vi "BeamProfiler.vi"() -> ()   [LabVIEW 2015]
uses:
  <vilib>/vision/Image Controls.llb/IMAQ Image.ctl
  <vilib>/userdefined/High Color/IMAQdx.ctl
  <vilib>/vision/driver/IMAQdx.llb/IMAQdx Buffer Number Mode.ctl
  <vilib>/vision/driver/IMAQdx.llb/IMAQdx Acquisition Mode.ctl
  <vilib>/vision/NI_Vision_Development_Module.lvlib
  <vilib>/vision/driver/NI_Vision_Acquisition_Software.lvlib
  <resource>/objmgr/imaqdx.rc
panel:
  out "Histogram Report 2":T1
  in  "Pixel Size":cluster{"X Step":sgl, "Y Step":sgl}={"X Step"=5.2, "Y Step"=5.2} {"Y Step" format="%.2f"; "X Step" format="%.2f"}
  out "Fit Pixel":dbl[](array[numeric])
  out "Ellipse Points":cluster{"x out":dbl, "y out":dbl}[](array[cluster])
  out "Cross lines":T2
  out "ROI Width":dbl
  out "Subsampling":i32(ring)=16 items=["1"=1, "2"=2, "4"=4, "8"=8, "16"=16]
  out "error Fitting":errorcluster
  out "GausFit Time":u32(graph)
  out "Gaus Param":T3(graph)
  in  "Rangefactor \n(multiple of w)":dbl=3.0
  out "Fitting error: Message":string
  out "parameter \narray":dbl[][](array[numeric])
  out "residue":dbl
  out "number of \nfunction calls":i32
  out "Fitting Time \n(ms)":u32
  in  "Gaussianfit":bool
  out "Image to fit":T4(plugin-control)
  in  "Tab Control":T5(tab)
  out "Histogramm of ROI":u32[](graph)
  out "Gray Level Intensities":T6 {"Standard  Deviation" format="%.2f"; "Mean Intensity" format="%.2f"; "Maximum Intensity" format="%.2f"; "Minimum Intensity" format="%.2f"}
  out "Sättigung":dbl format="%.2f %"
  out "3D Image 2":T4(plugin-control)
  in  "3D options":T7={"alpha"=15.0, "beta"=30.0, "border"=20, "background"=85, "plane"=2} {"beta" min=15 max=45 format="%.2f"; "alpha" min=15 max=45 format="%.2f"}
  out "Differece Image to Ideal Gaussian":T4(plugin-control)
  in  "DualZoom":bool
  in  "Show Difference Image":bool
  out "Minimal Value":sgl
  out "Maximal Value":sgl
  out "AbsDiff":T4(plugin-control)
  in  "Show Abs Difference Image":bool
  out "Histogram Diff ROI":T1 {"Standard  Variation" format="%.2f"; "Mean Value" format="%.2f"; "Interval Width" format="%.2f"; "Starting Value" format="%.2f"; "Maximal Value" format="%.2f"; "Minimal Value" format="%.2f"}
  out "Histogram Img ROI":T1 {"Standard  Variation" format="%.2f"; "Mean Value" format="%.2f"; "Interval Width" format="%.2f"; "Starting Value" format="%.2f"; "Maximal Value" format="%.2f"; "Minimal Value" format="%.2f"}
  out "Integrated Pixels":cluster{sgl, sgl}(graph)
  out "AbsDiff/Imag":sgl(graph)
  out "AbsDifference/ImageSum":sgl
  out "Integrated AbsDiff":sgl
  out "Integrated CamImage":sgl
  out "Recorded Background":T4(plugin-control)
  out "iValue\nChart":dbl(graph)
  in  "soll":dbl=220.0 min=10.0 max=240.0 step=1.0
  out "iValue":dbl
  in  "1/T":dbl=4.0
  out "ist":dbl
  out "ImgMax/Max":dbl
  in  "AutoAcquisitionState":T8(ring)
  in  "Next AEC & AGC\niteration":bool
  in  "Enable AEC & AGC":bool
  in  "Max Intensity":dbl=250.0 max=254.0
  out "Time\nAGC\nHist":dbl
  out "Time\nAGC/AEC\ncycle":dbl
  out "State":sgl(graph)
  in  "Gaussian Fit completed":bool
  out "Exit from Target Point":bool
  out "Beam Parameters Target Point":T9
  out "Target Point cross lines":T2
  out "Target Points Ellipse Points":cluster{"x out":dbl, "y out":dbl}[](array[cluster])
  in  "Set Target Point":bool
  in  "Show Target \nPoint Axes":bool
  out "Start StreamingLED":bool
  out "AcquisitionTime":dbl(graph)
  out "Time\nAcqisition(s)":dbl
  out "Time\nEvent(ms)":u32
  out "Histogram Report":T1
  out "Exit from AGC/AEC":bool
  out "ActValue:InverseExposure":dbl format="1 / %#_g ms"
  out "Image Busy":bool
  in  "Show Axes Overlay":bool=TRUE
  out "Exit from stream complete":bool
  out "Exit from Control refresh":bool
  out "Exit from Gaussian cycle":bool
  out "Exit from Eventloop":bool
  out "image heigth":u16
  out "image width":u16
  in  "Resolution":cluster{"X Step":u16, "Y Step":u16}={"X Step"=1280, "Y Step"=1024}
  out "IMAQ Actual Image":T4(plugin-control)
  out "GValueMin":dbl format="%#_4g"
  out "GValueMax":dbl format="%#_4g"
  out "EValueMin":dbl format="%#_4g"
  out "EValueMax":dbl format="%#_4g"
  out "error\nControl\nrefresh":errorcluster
  out "Buffer Number":u32
  out "Frame Rate":dbl(knob) scale=0.0..20.0
  out "ActVal:Gain":string
  out "ActValue:Exposure":string
  in  "Gain::Mode":u32(ring)=2 caption="Exposure::Mode" items=["Auto (Extended)", "Auto (Standard)", "Manual"]
  in  "Exposure::Mode":u32(ring)=2 items=["Auto (Extended)", "Auto (Standard)", "Manual"]
  in  "Set Gain":bool
  in  "Set Exposure":bool
  in  "Set: Gain::Value":i64 caption="Gain::Value" min=0 max=1728 step=16
  in  "Set: Exposure::Value":dbl=0.0625 caption="Exposure::Value" min=0.0001220703125 max=0.125
  out "Camera Handle":T10 caption="Session Out"
  in  "Camera Name":refnum<k21>="cam0" caption="IMAQdx Session"
  out "IMAQ Actual Image (RGB)":T4
  in  "Cyclic\nCalculation":bool=TRUE
  in  "Cycletime Task\nGaussian Fit":u32=1000
  out "Stream completed":bool
  in  "Stop Streaming":bool
  in  "Start Streaming":bool
  out "Stream error out":errorcluster
  out "Streaming Started":bool
  out "IMAQ Background Image":T4
  in  "Subtract Background":bool
  in  "Record Background":bool
  out "CAM\ninitialized":bool
  in  "Direction (NW)":T11(ring)
  in  "3D Image":bool
  in  "CalcHistogram":bool
  out "EventState":string
  out "error Event":errorcluster
  in  "error in":errorcluster
  in  "Start":bool
  in  "Tab Beam":enum32{"Beam Parameters", "Navigate to Target"}(tab)
  out "Beam Parameters":T9 {"Amplitude (Counts)" format="%#.2f"; "Position X (µm)" format="%.2f"; "Position Y (µm)" format="%.2f"; "Width 1 (µm)*" format="%.2f"; "Width 2 (µm)*" format="%.2f"; "Angle (°)" format="%.2f"; "Offset (Counts)" format="%.2f"}
  out "Mean \nRadius":dbl
  out "Ellipticity":dbl format="%#_3g"
  out "Point":T12 {"Y" format="%.2f"; "X" format="%.2f"}
  in  "Threshold (µm)":dbl=52.0
  out "dy":dbl
  out "dx":dbl
  out "left":bool
  out "down":bool
  out "up":bool
  out "right":bool
  out "center":bool
  out "Beam Parameters\nfor Target":T13
  out "Absolute Distance (µm)":dbl
  in  "stop":bool
  # "Shutdown"
  # "Overview: .\nRequirements: Vision Development Software, Vision Acquisition Software.\nInstructions: \n1. Select 'Camera Name',  'Resolution' and 'Pixel Size'\n2. Run the VI.\n3. Press 'Start'\n4. Pausing/Resuming Image with Start/Stop Streaming\n\nExit with 'Stop'"
  # "Aquisition Settings"
  # "ms"
  # "x /µm"
  # "y /µm"
  # "ms"
  # "Guess Pixel"
  # "Fit RAW"
  # "Fit Pixel"
  # "Fit µm"
  # "Amplitude"
  # "Position Mean X"
  # "Position Mean Y"
  # "Width 1 (1/e)"
  # "Width 2(1/e)"
  # "Orient. Angle"
  # "Offset"
  # "w(1/e) *sqrt(2) = w(1/e^2)"
  # "x"
  # "µm"
  # "Note: ROI has to be selected"
  # "Note: \nDifferent color scale"
  # "Background:\n1. Turn off subtraction\n2. Hide beam\n3. Take Image (Stream)\n4. Record background\nNote: not compatible \nwith AutoExposure"
  # "x"
  # "pixels"
  # "* Radius, 1/e^2, 13,5%, Width 1 > Width 2"
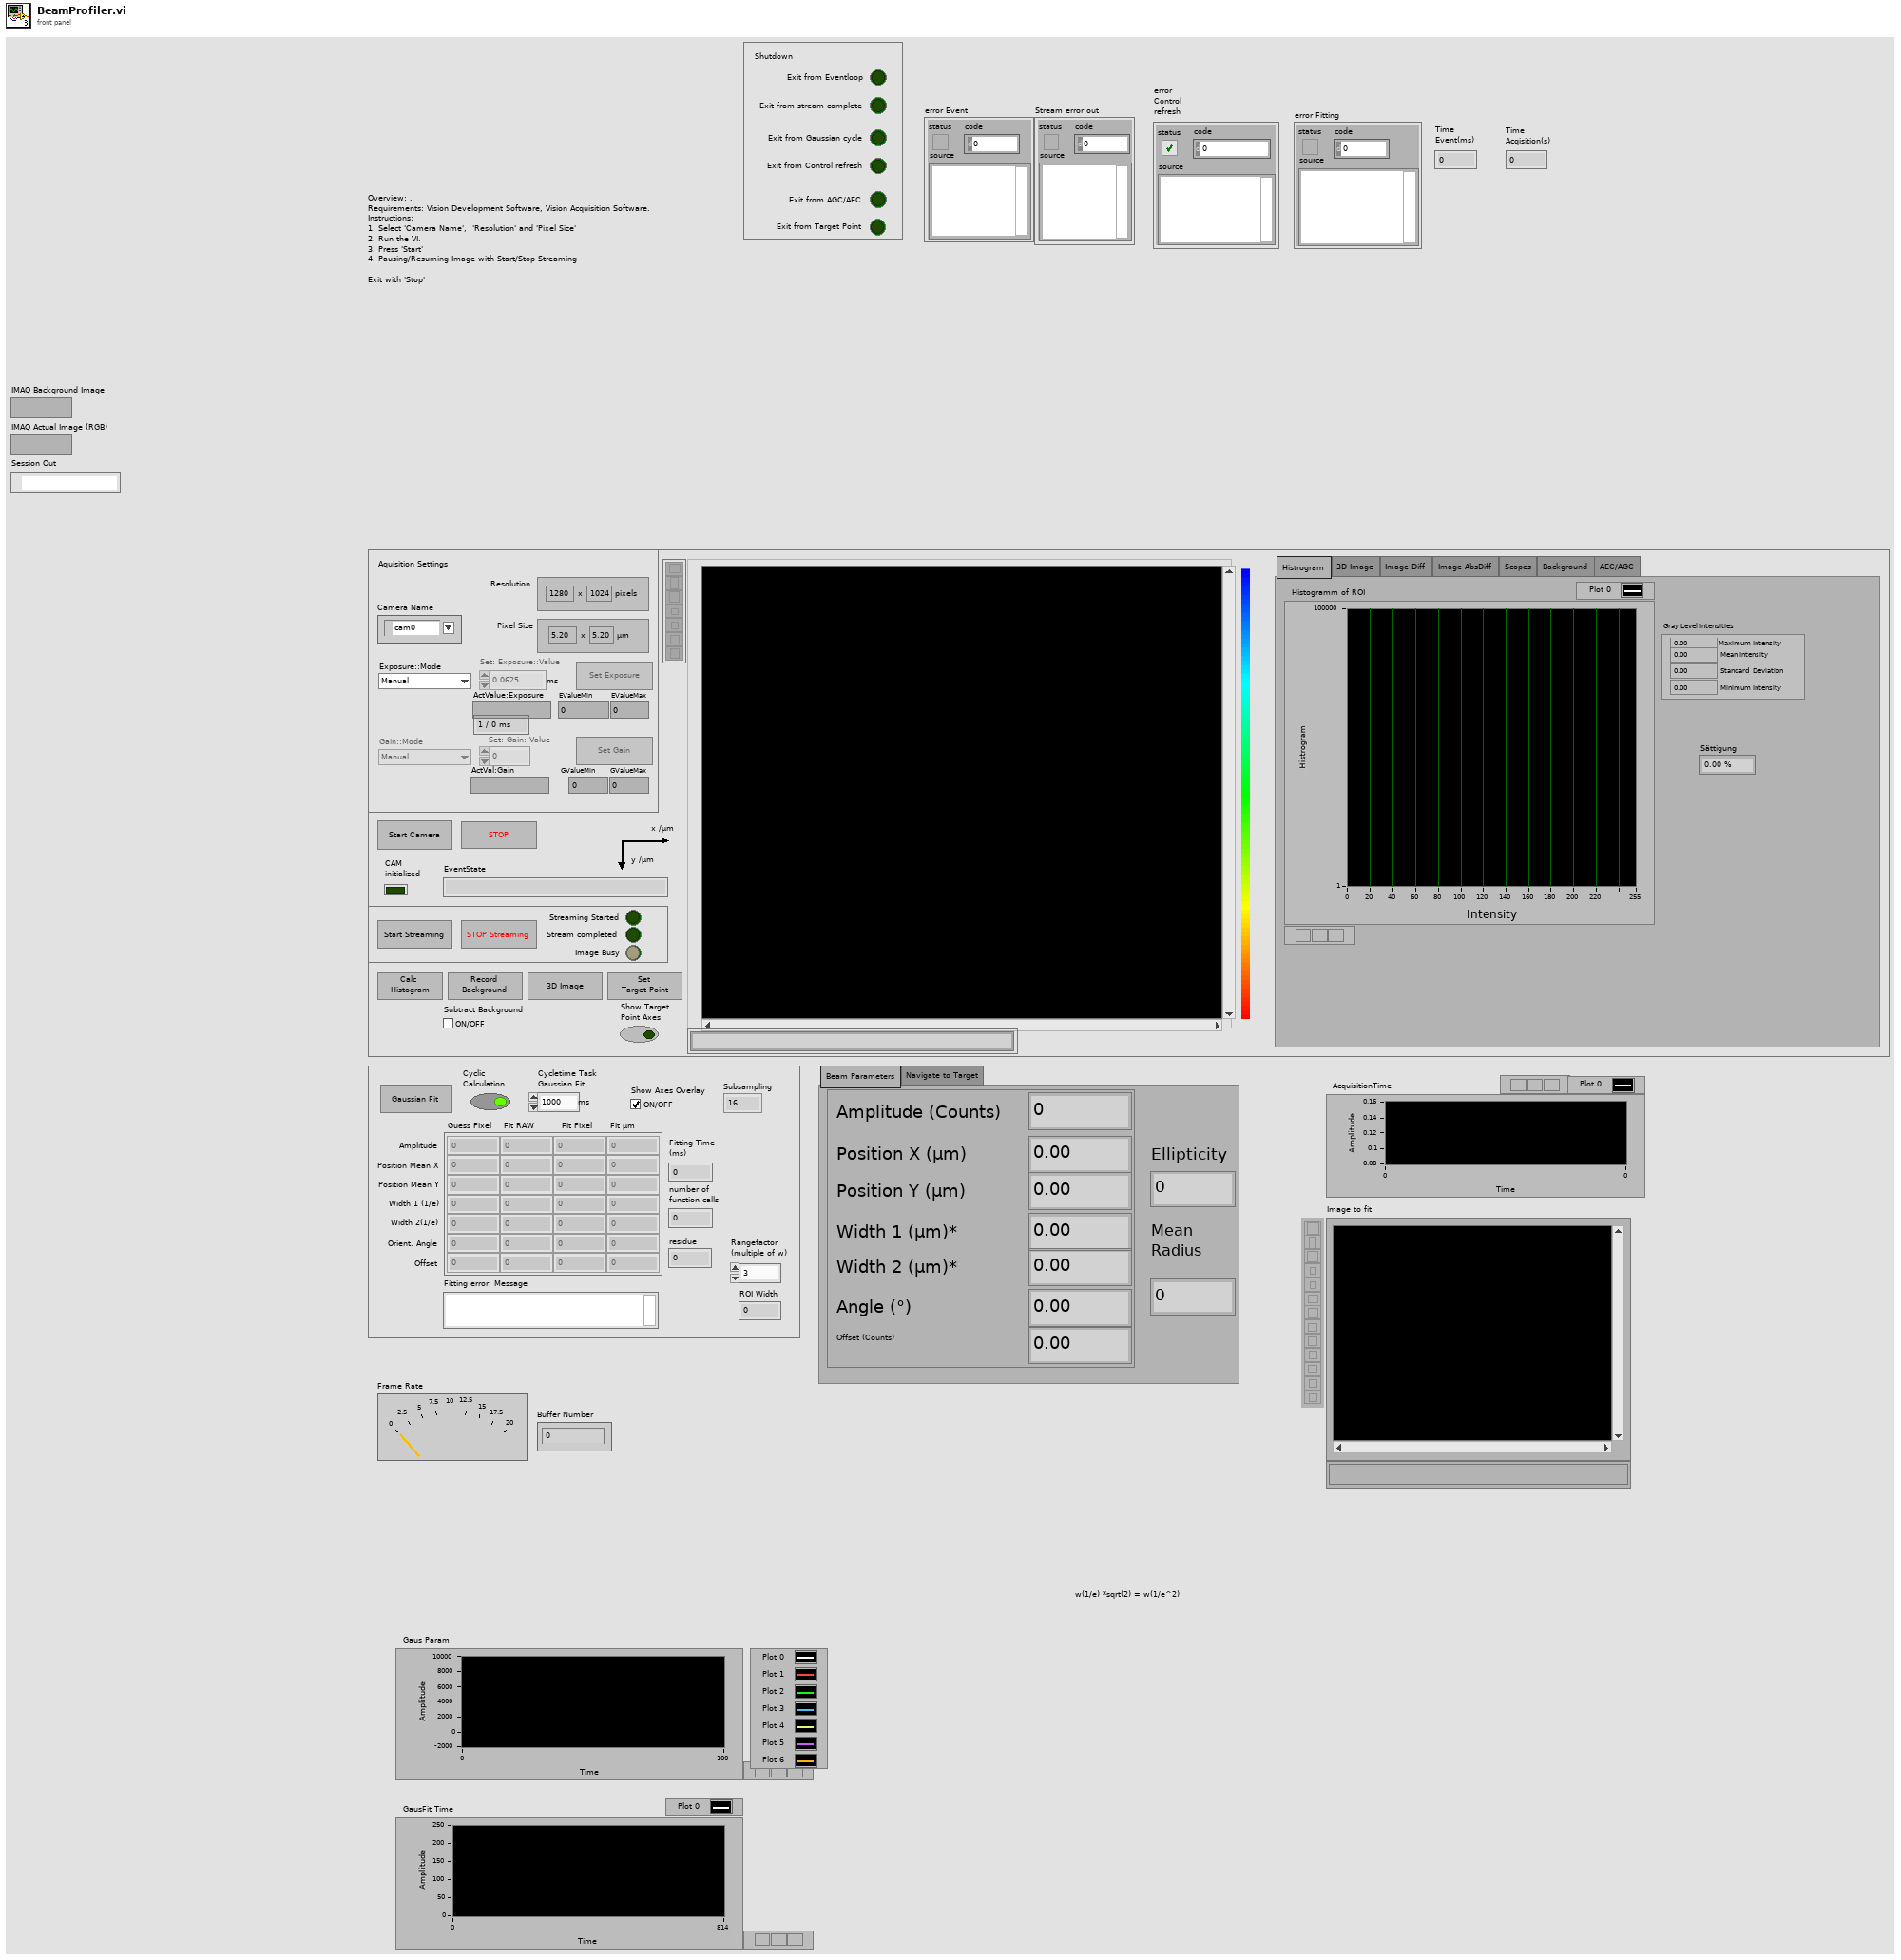
[diagram p1: front panel]
types:
  T1 = cluster{"histogram":u32[], "Minimal Value":sgl, "Maximal Value":sgl, "Starting Value":sgl, "Interval Width":sgl, "Mean Value":sgl, "Standard  Variation":sgl, "Area (pixels)":i32}
  T2 = cluster{"Line1 Start Point":cluster{"X":i32, "Y":i32}, "Line1 End Point":cluster{"X":i32, "Y":i32}, "Line2 Start Point":cluster{"X":i32, "Y":i32}, "Line2 End Point":cluster{"X":i32, "Y":i32}}
  T3 = cluster{"Amplitude (Counts)":dbl, "Position Max X(µm)":dbl, "Position Max Y(µm)":dbl, "Width 1 (µm)":dbl, "Width 2 (µm)":dbl, "Angle (°)":dbl, "Offset (Counts)":dbl}
  T4 = typedef "IMAQ Image.ctl" = refnum<image>
  T5 = enum32{"Histrogram", "3D Image", "Image Diff", "Image AbsDiff", "Scopes", "Background", "AEC/AGC"}
  T6 = cluster{"Mean Intensity":sgl, "Standard  Deviation":sgl, "Minimum Intensity":sgl, "Maximum Intensity":sgl}
  T7 = cluster{"alpha":sgl, "beta":sgl, "border":i32, "background":i32, "plane":i32}
  T8 = enum16{"idle", "init", "Wait before exposure", "Find max exposure", "Wait before gain", "Find max gain"}
  T9 = cluster{"Amplitude (Counts)":dbl, "Position X (µm)":dbl, "Position Y (µm)":dbl, "Width 1 (µm)*":dbl, "Width 2 (µm)*":dbl, "Angle (°)":dbl, "Offset (Counts)":dbl}
  T10 = typedef "IMAQdx.ctl" = refnum<k21>
  T11 = enum32{"North West", "South West", "South East", "North East"}
  T12 = typedef "IMAQ Point" = cluster{"X":sgl, "Y":sgl}
  T13 = cluster{"Amplitude (Counts)":dbl, "Position X (µm)":dbl, "Position Y (µm)":dbl}
  T14 = typedef "Image Type" = u32
  T15 = cluster{"Global Rectangle":i32[], "Contours":cluster{"Contour Type":u32, "ROI Type":u32, "Points":i32[]}[]}
  T16 = enum8{"Enabled", "Disabled", "Disabled and Grayed Out"}
  T17 = enum32{"Histrogram", "3D Image", "Image Diff", "Image AbsDiff", "Scopes", "Background"}
  T18 = typedef "NI_Vision_Acquisition_Software.lvlib/IMAQdx Acquisition Mode.ctl" = enum32{"One Shot", "Continuous"}
  T19 = cluster{"Amplitude (Counts)":dbl, "Position Max X(µm)":dbl, "Position Max Y(µm)":dbl}
  T20 = typedef "NI_Vision_Acquisition_Software.lvlib/IMAQdx Buffer Number Mode.ctl" = enum32{"Next", "Last", "Buffer Number", "Every", "Last New"}
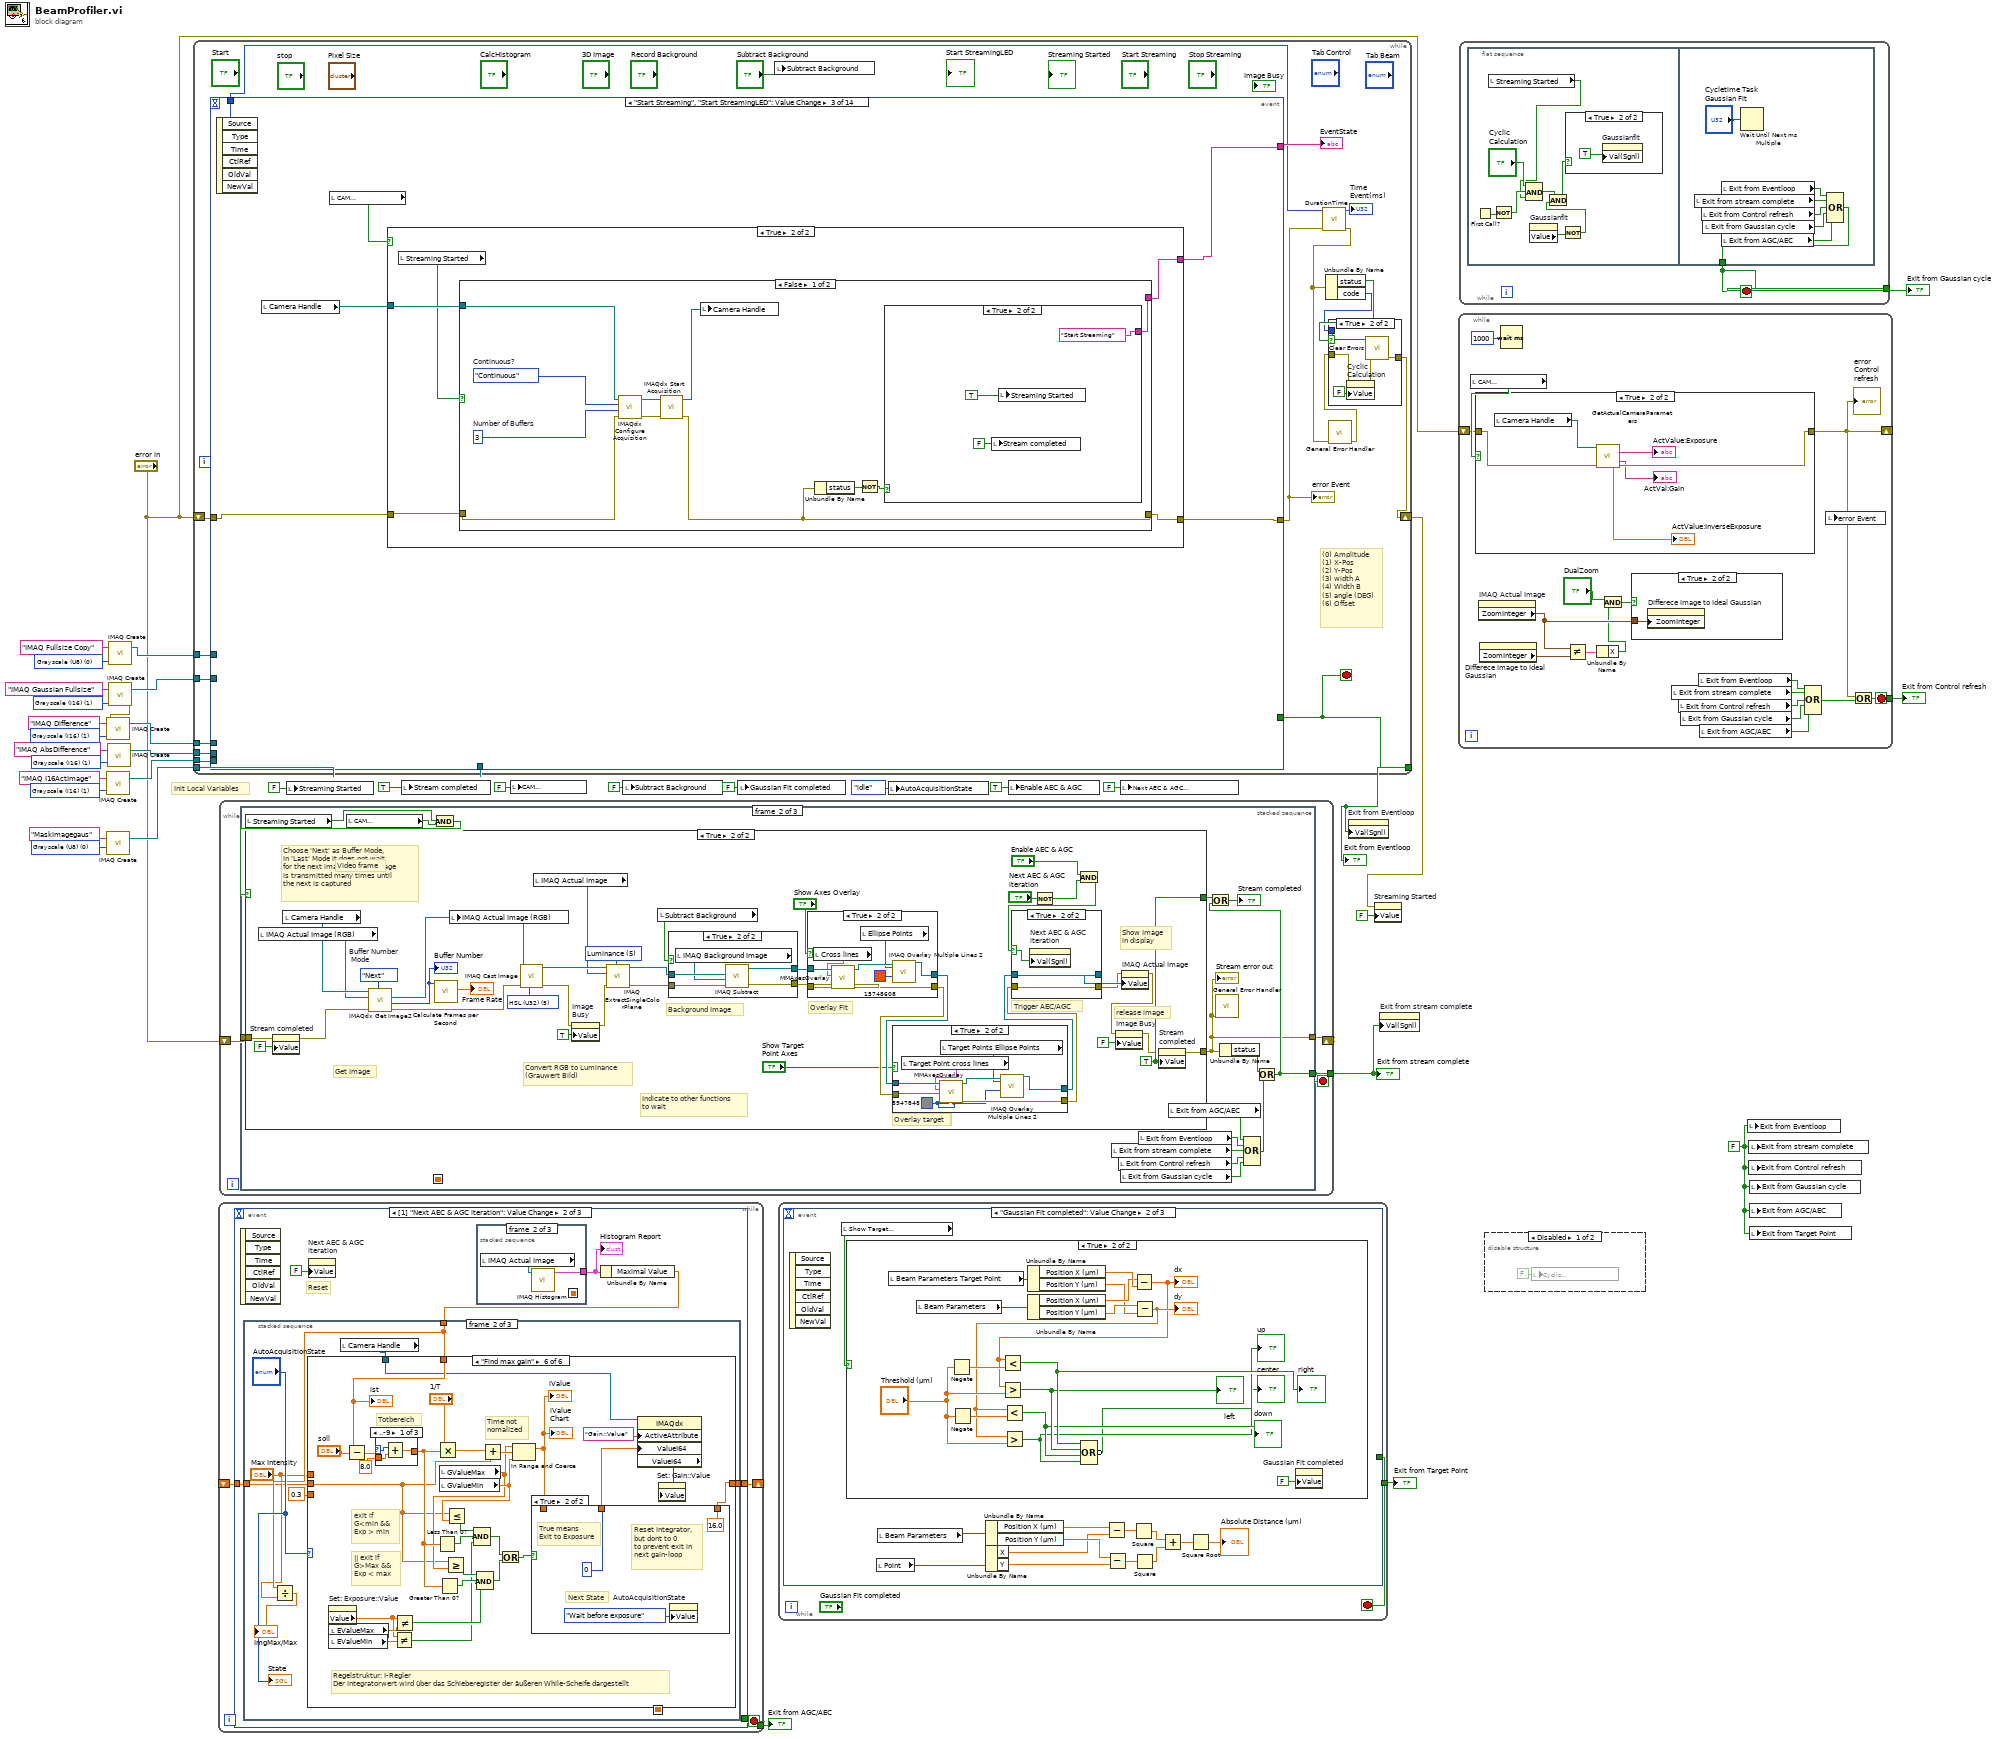
[diagram p0: block diagram]
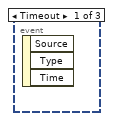
[diagram p2: hidden frame]
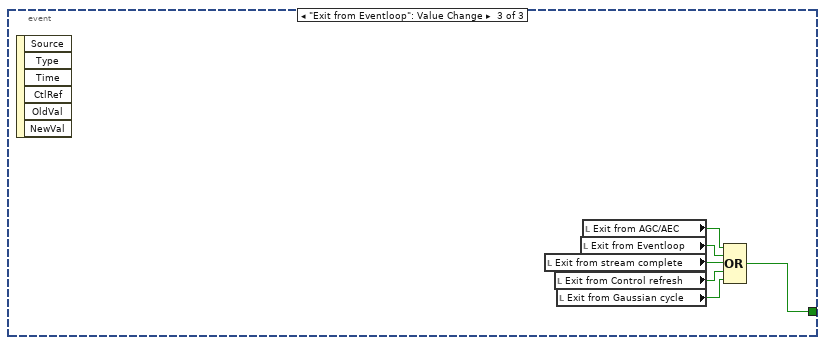
[diagram p4: hidden frame]
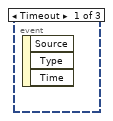
[diagram p6: hidden frame]
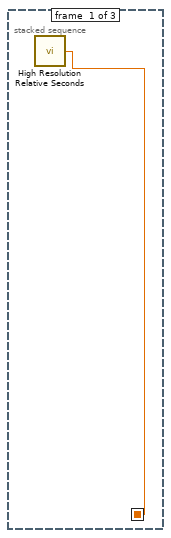
[diagram p7: hidden frame]
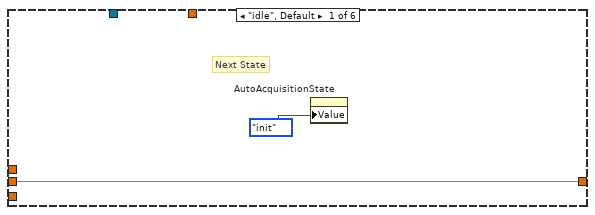
[diagram p8: hidden frame]
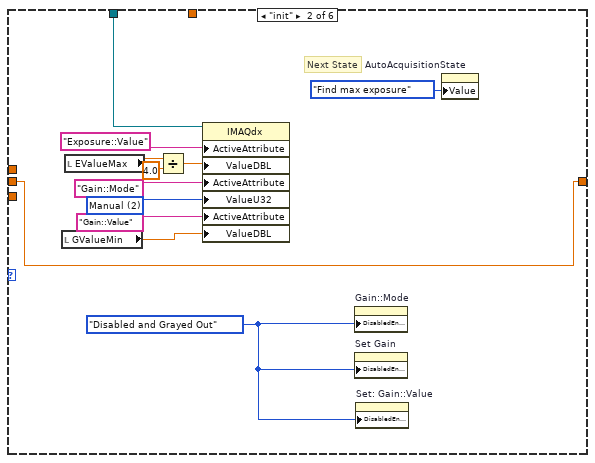
[diagram p9: hidden frame]
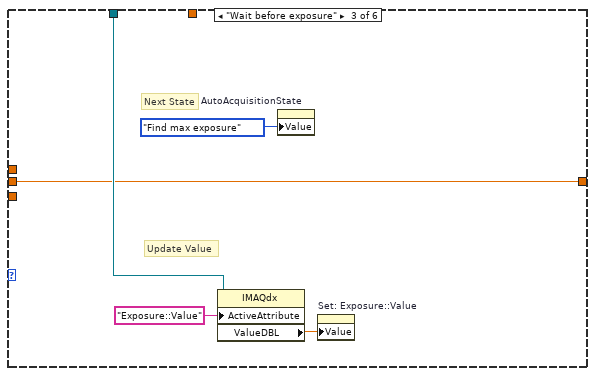
[diagram p10: hidden frame]
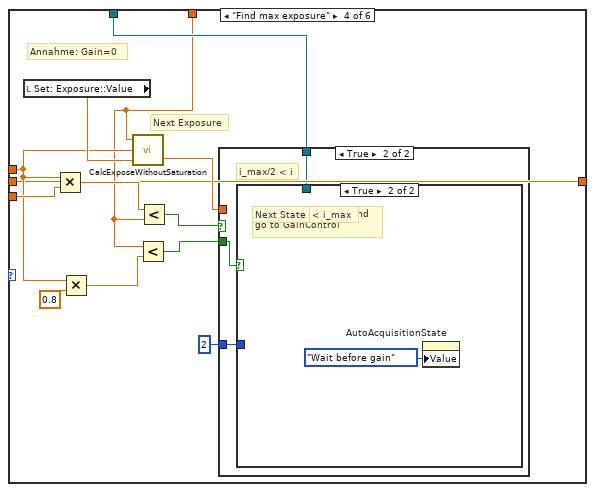
[diagram p11: hidden frame]
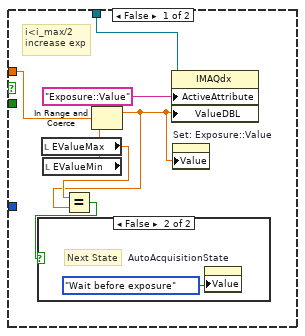
[diagram p12: hidden frame]
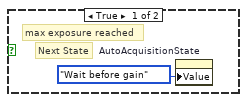
[diagram p13: hidden frame]
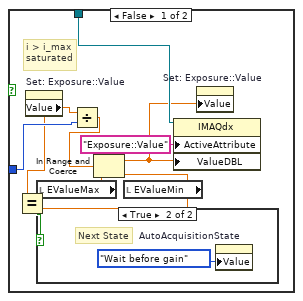
[diagram p14: hidden frame]
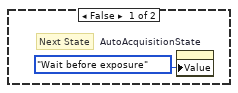
[diagram p15: hidden frame]
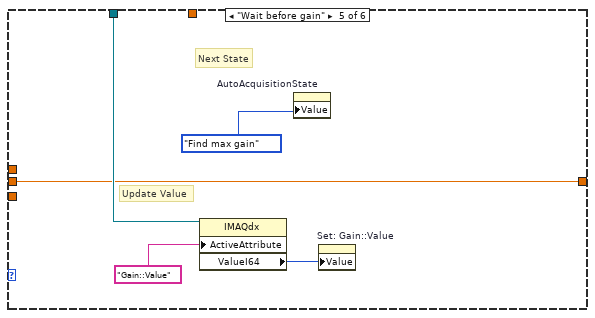
[diagram p16: hidden frame]
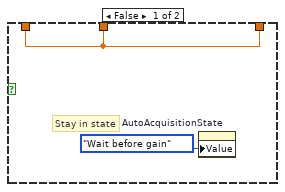
[diagram p17: hidden frame]
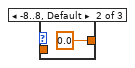
[diagram p18: hidden frame]
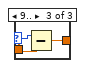
[diagram p19: hidden frame]
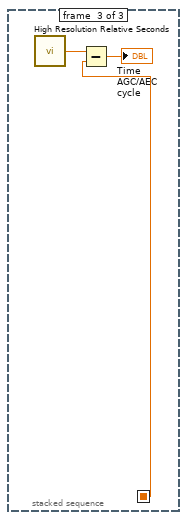
[diagram p20: hidden frame]
diagram:
  w3 = T14 0 items=["Grayscale (U8)", "Grayscale (I16)", "Grayscale (SGL)", "Complex (CSG)", "RGB (U32)", "HSL (U32)", "RGB (U64)", "Grayscale (U16)"] ("Image Type")
  w5 = T14 0 items=["Grayscale (U8)", "Grayscale (I16)", "Grayscale (SGL)", "Complex (CSG)", "RGB (U32)", "HSL (U32)", "RGB (U64)", "Grayscale (U16)"] ("Image Type")
  w9 = T14 1 items=["Grayscale (U8)", "Grayscale (I16)", "Grayscale (SGL)", "Complex (CSG)", "RGB (U32)", "HSL (U32)", "RGB (U64)", "Grayscale (U16)"] ("Image Type")
  w20 = T14 1 items=["Grayscale (U8)", "Grayscale (I16)", "Grayscale (SGL)", "Complex (CSG)", "RGB (U32)", "HSL (U32)", "RGB (U64)", "Grayscale (U16)"] ("Image Type")
  w16 = T14 1 items=["Grayscale (U8)", "Grayscale (I16)", "Grayscale (SGL)", "Complex (CSG)", "RGB (U32)", "HSL (U32)", "RGB (U64)", "Grayscale (U16)"] ("Image Type")
  w15 = T14 1 items=["Grayscale (U8)", "Grayscale (I16)", "Grayscale (SGL)", "Complex (CSG)", "RGB (U32)", "HSL (U32)", "RGB (U64)", "Grayscale (U16)"] ("Image Type")
  w22 = FALSE ("Gaussianfit")
  # "Init Local Variables"
  n1 = call "IMAQ Create"("Image Name"="IMAQ I16ActImage", "Image Type"=w9) -> ("New Image"=w8:T4)  [unwired: 3 in, 1 out]
  n2 = call "IMAQ Create"("Image Name"="MaskImagegaus", "Image Type"=w5) -> ("New Image"=w6:T4)  [unwired: 3 in, 1 out]
  n3 = call "IMAQ Create"("Image Name"="IMAQ AbsDifference", "Image Type"=w20) -> ("New Image"=w11:T4)  [unwired: 3 in, 1 out]
  n4 = call "IMAQ Create"("Image Name"="IMAQ Gaussian Fullsize", "Image Type"=w15) -> ("New Image"=w13:T4, "error out"=w18:errorcluster)  [unwired: 3 in]
  n5 = call "IMAQ Create"("Image Name"="IMAQ Difference", "Image Type"=w16, "error in (no error)"=w18) -> ("New Image"=w12:T4)  [unwired: 2 in, 1 out]
  n6 = call "IMAQ Create"("Image Name"="IMAQ Fullsize Copy", "Image Type"=w3) -> ("New Image"=w2:T4)  [unwired: 3 in, 1 out]
  n7 = while {
    shift-right: [w51] -> w33
    shift-left: "error in" -> [w53]
    tunnel: [w39] -> w27
    tunnel: w13 -> [w44]
    tunnel: w12 -> [w43]
    tunnel: w11 -> [w42]
    tunnel: w8 -> [w41]
    tunnel: w6 -> [w38]
    tunnel: w2 -> [w40]
    stop <- w39 stop-if-true
    # "(0) Amplitude\n(1) X-Pos\n(2) Y-Pos\n(3) width A\n(4) Width B\n(5) angle (DEG)\n(6) Offset"
    n8 = event shown="[2] \"Start Streaming\", \"Start StreamingLED\": Value Change" {
      selector: _ -> [_ _ _ _ _ _ _ _ _ _ _ _ _ _]
      dyn-events: _ -> [_ _ _ _ _ _ _ _ _ _ _ _ _ _]
      timeout: _ -> [_ _ _ _ _ _ _ _ _ _ _ _ _ _]
      tunnel: [_ _ _ _ _ _ _ _ _ _ _ w512 _ _] -> w39
      tunnel: [_ w68 w114 w149 w222 w319 w337 w353 w393 w429 w456 w514 w562 _] -> w45
      tunnel: ["Timeout" ("MainState") w66 w113 w148 _ w320 w336 w350 w390 w427 w457 w508 w561 _] -> w55
      tunnel: w53 -> [_ w65 w112 _ w209 w322 w338 w354 w394 w428 w455 w507 w565 _]
      tunnel: [w62 w64 w111 w141 w212 w318 w334 w352 w392 w426 w454 w506 w564 _] -> w49
      tunnel: w44 -> [_ _ _ _ w189 _ _ _ _ _ _ _ _ _]
      tunnel: w43 -> [_ _ _ _ w185 _ _ _ _ _ _ _ _ _]
      tunnel: w42 -> [_ _ _ _ w186 _ _ _ _ _ _ _ _ _]
      tunnel: w41 -> [_ _ _ _ w187 _ _ _ _ _ _ _ _ _]
      tunnel: w40 -> [_ _ _ _ w234 _ _ _ _ _ _ _ _ _]
      tunnel: w38 -> [_ _ _ _ w188 _ _ _ _ _ _ _ _ _]
      event Timeout {
        n9 = event-data() -> ("Time"=w62:u32)  [unwired: 1 in, 2 out]
      }
      event "Start": Value Change {
        n10 = event-data() -> ("Time"=w64:u32)  [unwired: 1 in, 5 out]
        n11 = local read "CAM\ninitialized"() -> (w67:bool)
        n12 = case shown="False" w67 {
          tunnel: [w86 w109] -> w68
          tunnel: ["Camera starting" ("MainState") "Camera already started" ("MainState")] -> w66
          tunnel: w65 -> [w90 w109]
          frame False {
            w87 = T14 0 items=["Grayscale (U8)", "Grayscale (I16)", "Grayscale (SGL)", "Complex (CSG)", "RGB (U32)", "HSL (U32)", "RGB (U64)"] ("Image Type")
            w94 = T14 0 items=["Grayscale (U8)", "Grayscale (I16)", "Grayscale (SGL)", "Complex (CSG)", "RGB (U32)", "HSL (U32)", "RGB (U64)"] ("Image Type")
            w96 = T14 0 items=["Grayscale (U8)", "Grayscale (I16)", "Grayscale (SGL)", "Complex (CSG)", "RGB (U32)", "HSL (U32)", "RGB (U64)", "Grayscale (U16)"] ("Image Type")
            n13 = Unbundle By Name("Resolution") -> ("X Step"=→"image width":u16, "Y Step"=→"image heigth":u16)
            n14 = call <vilib>:"IMAQdx Open Camera.vi"("error in"=w90, "Session In"="Camera Name") -> ("error out"=w89:errorcluster, "Session Out"=w85:T10)  [unwired: 1 in, 7 out]
            "Camera Handle" <- w85
            n15 = call "IMAQ Create"("Image Name"="Actual Image", "Image Type"=w96, "error in (no error)"=w89) -> ("New Image"=w78:T4, "error out"=w92:errorcluster)  [unwired: 2 in]
            "IMAQ Actual Image" <- w78
            n16 = call "IMAQ Create"("Image Name"="Actual Image (RGB)", "Image Type"=w94, "error in (no error)"=w92) -> ("New Image"=w93:T4, "error out"=w91:errorcluster)  [unwired: 2 in]
            "IMAQ Actual Image (RGB)" <- w93
            n17 = call "IMAQ Create"("Image Name"="Background Image", "Image Type"=w87, "error in (no error)"=w91) -> ("New Image"=w99:T4, "error out"=w81:errorcluster)  [unwired: 2 in]
            "IMAQ Background Image" <- w99
            n18 = local write "Camera Handle"(w85) -> ()
            n19 = local write "IMAQ Actual Image (RGB)"(w93) -> ()
            n20 = local write "IMAQ Background Image"(w99) -> ()
            n21 = local write "IMAQ Actual Image"(w78) -> ()
            n22 = disable-structure shown="Enabled" {
              disable-tunnel: w81 -> [w107 _]
              disable-tunnel: [w106 _] -> w80
              frame Enabled {
                w105 = u32 0 items=["Auto (Extended)", "Auto (Standard)", "Manual"] ("Gain::Mode")
                n23 = property on="Exposure::Mode" class="Ring (strict)"(error in=w107, "Val(Sgnl)"=w105) -> (error out=w108:errorcluster)  [unwired: 1 in, 1 out]
                n24 = property on="Gain::Mode" class="Ring (strict)"(error in=w108, "Val(Sgnl)"=w105) -> (error out=w106:errorcluster)  [unwired: 1 in, 1 out]
              }
              frame Disabled {
              }
            }
            n25 = property class="IMAQdx"(reference=w85, error in=w80, "ActiveAttribute"="Exposure::Value", "ActiveAttribute"="Gain::Value") -> (error out=w86:errorcluster, "ValueDBL"=w83:dbl, "MinDBL"=w74:dbl, "MaxDBL"=w73:dbl, "ValueI64"=w79:i64, "MinDBL"=w72:dbl, "MaxDBL"=w71:dbl)  [unwired: 1 out]
            "EValueMin" <- w74
            "EValueMax" <- w73
            "GValueMin" <- w72
            "GValueMax" <- w71
            n26 = property on="Set: Exposure::Value" class="DigNum (strict)"("Value"=w83) -> ()  [unwired: 2 in, 2 out]
            n27 = property on="Set: Gain::Value" class="DigNum (strict)"("Value"=w79) -> ()  [unwired: 2 in, 2 out]
            n28 = property on="Set: Gain::Value" class="DigNum (strict)"("Maximum"=w71, "Minimum"=w72) -> ()  [unwired: 2 in, 2 out]
            n29 = property on="Set: Exposure::Value" class="DigNum (strict)"("Minimum"=w74, "Maximum"=w73) -> ()  [unwired: 2 in, 2 out]
            n30 = Unbundle By Name(w86) -> ("status"=w98:bool)
            n31 = Not(x=w98) -> (.not. x?=w97:bool)
            n32 = Or(x=TRUE, y=w97) -> (x .or. y?=→"CAM\ninitialized":bool)
            n33 = property on="Start StreamingLED" class="Bool (strict)"() -> ("Value"=w70:bool)  [unwired: 2 in, 2 out]
            n34 = Not(x=w70) -> (.not. x?=w69:bool)
            n35 = property on="Start StreamingLED" class="Bool (strict)"("Val(Sgnl)"=w69) -> ()  [unwired: 2 in, 2 out]
          }
          frame True {
          }
        }
      }
      event "Start Streaming", "Start StreamingLED": Value Change {
        n36 = event-data() -> ("Time"=w111:u32)  [unwired: 1 in, 5 out]
        n37 = local read "Camera Handle"() -> (w116:T10)
        n38 = local read "CAM\ninitialized"() -> (w115:bool)
        n39 = case shown="True" w115 {
          tunnel: w116 -> [_ w122]
          tunnel: w112 -> [w118 w121]
          tunnel: [w118 w120] -> w114
          tunnel: ["Camera not initialized, Press Start Camera" ("MainState") w123] -> w113
          frame False {
            n40 = call "Display Message to User2"() -> ()  [unwired: 10 in, 2 out]
          }
          frame True {
            n41 = local read "Streaming Started"() -> (w119:bool)
            n42 = case shown="False" w119 {
              tunnel: [w132 "Stream already started" ("MainState")] -> w123
              tunnel: w122 -> [w129 _]
              tunnel: w121 -> [w126 w139]
              tunnel: [w125 w139] -> w120
              frame False {
                w127 = u32 3  # Number of Buffers
                w128 = IMAQdx_Acquisition_Mode."Continuous"  # Continuous?
                n43 = call <vilib>:"IMAQdx Configure Acquisition.vi"("error in"=w126, "Number of Buffers"=w127, "Continuous?"=w128, "Session In"=w129) -> ("error out"=w131:errorcluster, "Session Out"=w130:T10)  [unwired: 6 out]
                n44 = call <vilib>:"IMAQdx Start Acquisition.vi"("error in"=w131, "Session In"=w130) -> ("error out"=w125:errorcluster, "Session Out"=w124:T10)  [unwired: 8 out]
                n45 = local write "Camera Handle"(w124) -> ()
                n46 = Unbundle By Name(w125) -> ("status"=w134:bool)
                n47 = Not(x=w134) -> (.not. x?=w133:bool)
                n48 = case shown="True" w133 {
                  tunnel: ["Error while starting stream" ("MainState") "Start Streaming" ("MainState")] -> w132
                  frame False {
                  }
                  frame True {
                    n49 = local write "Stream completed"(FALSE ("Stream completed")) -> ()
                    n50 = local write "Streaming Started"(TRUE ("Stream Start")) -> ()
                  }
                }
              }
              frame True {
              }
            }
          }
        }
      }
      event "Stop Streaming": Value Change {
        n51 = event-data() -> ("Time"=w141:u32)  [unwired: 1 in, 5 out]
        n52 = local read "Streaming Started"() -> (w151:bool)
        n53 = local read "Camera Handle"() -> (w152:T10)
        n54 = local read "error Event"() -> (w150:errorcluster)
        n55 = flat-sequence {
          tunnel: w150 -> [w154]
          tunnel: w151 -> [w155]
          tunnel: w152 -> [w156]
          tunnel: [w156] -> w147
          tunnel: [w155] -> w145
          tunnel: [w154] -> w143
          tunnel: w147 -> [w160]
          tunnel: [w160] -> w146
          tunnel: w145 -> [w159]
          tunnel: [w159] -> w144
          tunnel: w143 -> [w158]
          tunnel: [w158] -> w142
          tunnel: [w169] -> w149
          tunnel: [w168] -> w148
          tunnel: w146 -> [w172]
          tunnel: w144 -> [w171]
          tunnel: w142 -> [w170]
          frame #0 {
            n56 = local write "Streaming Started"(FALSE ("Streaming Started")) -> ()
          }
          frame #1 {
            # "With Timeout"
            n57 = Tick Count (ms)() -> (millisecond timer value=w157:u32)
            n58 = while {
              tunnel: w157 -> [w166]
              stop <- w161 stop-if-true
              n59 = local read "Stream completed"() -> (w162:bool)
              n60 = Tick Count (ms)() -> (millisecond timer value=w167:u32)
              n61 = Subtract(x=w167, y=w166) -> (x-y=w165:u32)
              n62 = Greater?(x=w165, y=u32 2000) -> (0:w163:bool)
              n63 = Or(x=w162, y=w163) -> (x .or. y?=w161:bool)
            }
          }
          frame #2 {
            n64 = case shown="True" w171 {
              tunnel: w172 -> [_ w176]
              tunnel: w170 -> [w174 w178]
              tunnel: [w174 w177] -> w169
              tunnel: ["no stream running" ("MainState") "stream stopped" ("MainState")] -> w168
              frame False {
              }
              frame True {
                n65 = call <vilib>:"IMAQdx Stop Acquisition.vi"("error in"=w178, "Session In"=w176) -> ("error out"=w179:errorcluster, "Session Out"=w180:T10)  [unwired: 8 out]
                n66 = call <vilib>:"IMAQdx Unconfigure Acquisition.vi"("error in"=w179, "Session In"=w180) -> ("error out"=w177:errorcluster, "Session Out"=w175:T10)  [unwired: 8 out]
                n67 = local write "Camera Handle"(w175) -> ()
              }
            }
          }
        }
      }
      event "Gaussianfit": Value Change {
        # "Der Fehler wird gesondert\nangzeigt und nach einem \nZyklus gelöscht"
        # "Difference Image"
        # "Todo: Possibility to deactivate AutoRoi"
        # "Previous"
        # "Indicator for Target finding \ncycle"
        n68 = event-data() -> ("Time"=w212:u32)  [unwired: 1 in, 5 out]
        n69 = Or(x="Show Difference Image", y="Show Abs Difference Image") -> (x .or. y?=w184:bool)
        n70 = flat-sequence {
          tunnel: w234 -> [w317]
          tunnel: w233 -> [w316]
          tunnel: [w315] -> w217
          tunnel: w209 -> [w314]
          tunnel: [w313] -> w208
          frame #0 {
            n71 = while {
              stop <- w312 continue-if-true
              n72 = property on="Image Busy" class="Bool (strict)"() -> ("Value"=w312:bool)  [unwired: 2 in, 2 out]
            }
          }
          frame #1 {
            n73 = call "IMAQ Copy"("error in (no error)"=w314, "Image Dst"=w317, "Image Src"=w316) -> ("error out"=w313:errorcluster, "Image Dst Out"=w315:T4)  [unwired: 3 in]
          }
        }
        n74 = local read "IMAQ Actual Image"() -> (w233:T4)
        n75 = local read "error Fitting"() -> (w195:errorcluster)
        n76 = local read "residue"() -> (w199:dbl)
        n77 = local read "Fit Pixel"() -> (w197:dbl[])
        n78 = Unbundle By Name(w195) -> ("status"=w194:bool, "code"=w196:i32)
        n79 = case shown="True" w194 {
          tunnel: w196 -> [_ w300]
          tunnel: w195 -> [_ w299]
          frame False {
          }
          frame True {
            n80 = call <vilib>:"Clear Errors.vi"("error in (no error)"=w299, "specific error code to clear (0: all)"=w300) -> ()  [unwired: 4 in, 2 out]
          }
        }
        n81 = First Call?() -> (First Call?: T/F=w201:bool)
        n82 = Equal To 0?(x=w199) -> (x = 0?=w200:bool)
        n83 = Greater?(x=w199, y=100.0) -> (0:w202:bool)
        n84 = local read "Resolution"() -> (w193:cluster{"X Step":u16, "Y Step":u16})
        n85 = Compound Arithmetic op=OR(w202, w200, w201, w194) -> (w198:bool)
        n86 = case shown="True" w198 {
          tunnel: [w302 w306] -> w190
          tunnel: w217 -> [_ w305]
          tunnel: w208 -> [w301 w304]
          tunnel: [w301 w303] -> w207
          tunnel: w197 -> [w302 _]
          frame False {
          }
          frame True {
            n87 = call "ParameterGuess.vi"("error in"=w304, "Image IN"=w305) -> ("error out"=w303:errorcluster, "best fit parameters OUT"=w306:dbl[])  [unwired: 8 in]
          }
        }
        n88 = case shown="True" w184 {
          tunnel: w190 -> [_ w273]
          tunnel: w189 -> [_ w272]
          tunnel: w187 -> [_ w271]
          tunnel: w188 -> [_ w269]
          tunnel: w186 -> [_ w267]
          tunnel: w185 -> [_ w266]
          tunnel: "Show Abs Difference Image" -> [_ w259]
          frame False {
          }
          frame True {
            w270 = T14 1 items=["Grayscale (U8)", "Grayscale (I16)", "Grayscale (SGL)", "Complex (CSG)", "RGB (U32)", "HSL (U32)", "RGB (U64)", "Grayscale (U16)"] ("Image Type")
            n89 = local read "IMAQ Actual Image"() -> (w268:T4)
            n90 = local read "Resolution"() -> (w264:cluster{"X Step":u16, "Y Step":u16})
            n91 = call "IMAQ Cast Image"("Image Type"=w270, "Image Dst"=w271, "Image Src"=w268) -> ("Image Dst Out"=w265:T4)  [unwired: 7 in, 1 out]
            n92 = call "GenerateGaussianBeamImage.vi"("Image Resolution"=w264, "Fits Pixel"=w273, "Image"=w272) -> ("Gaussian Surface Image"=w263:T4)  [unwired: 7 in, 1 out]
            n93 = case shown="True" w259 {
              tunnel: w269 -> [_ w287]
              tunnel: w268 -> [_ w285]
              tunnel: w267 -> [_ w282]
              tunnel: w265 -> [_ w281]
              tunnel: w263 -> [_ w275]
              frame False {
              }
              frame True {
                # "Empty Roi"
                n94 = control-ref of="IMAQ Actual Image"() -> (w288:refnum<vi>)
                n95 = property class="ImageControl"(reference=w288) -> ("ROI"=w277:T15)  [unwired: 1 in, 2 out]
                n96 = Unbundle By Name(w277) -> ("Global Rectangle"=w279:i32[])  [unwired: 1 out]
                n97 = Array Size(array=w279) -> (size(s)=w280:i32)
                n98 = Equal To 0?(x=w280) -> (x = 0?=w278:bool)
                n99 = case shown="True" w278 {
                  tunnel: [w297 T15 {"Global Rectangle"=[0, 0, 1280, 1024], "Contours"=[{"Contour Type"=0, "ROI Type"=3, "Points"=[0, 0, 1279, 1023]}]} ("ROI")] -> w276
                  tunnel: w277 -> [w297 _]
                  frame False {
                  }
                  frame True {
                  }
                }
                n100 = call "IMAQ Absolute Difference"("Image Src A"=w281, "Image Dst"=w282, "Image Src B"=w275) -> ("Image Dst Out"=w274:T4)  [unwired: 4 in, 1 out]
                "AbsDiff" <- w274
                n101 = call "IMAQ ROIToMask 2"("ROI Descriptor"=w276, "Image"=w287) -> ("Image Out"=w284:T4)  [unwired: 7 in, 2 out]
                n102 = call "IMAQ Histogram"("Image Mask"=w284, "Image"=w274) -> ("Histogram Report"=w286:T1)  [unwired: 8 in, 1 out]
                "Histogram Diff ROI" <- w286
                n103 = call "IMAQ Histogram"("Image Mask"=w284, "Image"=w285) -> ("Histogram Report"=w283:T1)  [unwired: 8 in, 1 out]
                "Histogram Img ROI" <- w283
                n104 = Unbundle By Name(w286) -> ("Mean Value"=w296:sgl, "Area (pixels)"=w295:i32)
                n105 = Unbundle By Name(w283) -> ("Mean Value"=w294:sgl, "Area (pixels)"=w293:i32)
                n106 = Divide(x=w296, y=w294) -> (x/y=→"AbsDifference/ImageSum" →"AbsDiff/Imag":sgl)
                n107 = Multiply(x=w296, y=w295) -> (x*y=w292:sgl)
                "Integrated AbsDiff" <- w292
                n108 = Multiply(x=w294, y=w293) -> (x*y=w291:sgl)
                "Integrated CamImage" <- w291
                n109 = Bundle(w292, w291) -> (→"Integrated Pixels":cluster{sgl, sgl})  [unwired: 1 in]
              }
            }
            n110 = call "IMAQ Subtract"("Image Src A"=w265, "Image Dst"=w266, "Image Src B"=w263) -> ("Image Dst Out"=w258:T4)  [unwired: 4 in, 1 out]
            n111 = local read "Ellipse Points"() -> (w256:cluster{"x out":dbl, "y out":dbl}[])
            n112 = call "IMAQ Overlay Multiple Lines 2"("Image"=w258, "Line End Points"=w256, "Color"=u32 15748608) -> ("Image Out"=→"Differece Image to Ideal Gaussian":T4)  [unwired: 11 in, 1 out]
            n113 = call "IMAQ Histogram"("Image"=w258) -> ("Histogram Report"=w262:T1)  [unwired: 9 in, 1 out]
            "Histogram Report 2" <- w262
            n114 = Unbundle By Name(w262) -> ("Minimal Value"=→"Minimal Value":sgl, "Maximal Value"=→"Maximal Value":sgl)
          }
        }
        n115 = call "ROIAroundGaussian.vi"("Resolution"=w193, "Rangefactor (multiple w)"="Rangefactor \n(multiple of w)", "Fit Pixel"=w190) -> ("Subsampling"=w192:i32, "ROI Offset"=w220:i32[], "ROI"=w232:T15, "ROI Width"=→"ROI Width":dbl, "Rectangle (Array)"=w182:i32[])  [unwired: 3 in, 1 out]
        "Subsampling" <- w192
        n116 = property on="IMAQ Actual Image" class="ImageControl"("ROI"=w232) -> ()  [unwired: 2 in, 2 out]
        n117 = call "IMAQ Extract 2"("Y Step Size"=w192, "Optional Rectangle"=w182, "error in (no error)"=w207, "X Step Size"=w192, "Image Dst"=w217, "Image Src"=w217) -> ("error out"=w206:errorcluster, "Image Dst Out"=w214:T4)  [unwired: 4 in]
        "Image to fit" <- w214
        n118 = call "FitParametersPixel2RAW.vi"("Subsampling"=w192, "ROI Offset"=w220, "Fits Pixel"=w190) -> ("Fit RAW"=w219:dbl[])  [unwired: 8 in]
        n119 = local read "CAM\ninitialized"() -> (w254:bool)
        n120 = call "IMAQ ImageToArray"("error in (no error)"=w206, "Image"=w214) -> ("error out"=w204:errorcluster, "Image Pixels (U8)"=w231:u8[][])  [unwired: 2 in, 3 out]
        n121 = Transpose 2D Array(2D array=w231) -> (transposed array=w218:u8[][])
        n122 = Not(x=w254) -> (.not. x?=w230:bool)
        n123 = call "fit3.vi"("image array"=w218, "estimated parameters"=w219, "error in (no error)"=w204, "disable fit"=w230) -> ("number of function calls"=→"number of \nfunction calls":i32, "Fitting Time"=→"Fitting Time \n(ms)":u32, "best fit parameters"=w226:dbl[], "residue"=→"residue":dbl, "error out"=w221:errorcluster)  [unwired: 6 in, 1 out]
        "error Fitting" <- w221
        n124 = Unbundle By Name(w221) -> ("source"=→"Fitting error: Message":string)
        n125 = local read "IMAQ Actual Image"() -> (w245:T4)
        n126 = local read "Pixel Size"() -> (w251:cluster{"X Step":sgl, "Y Step":sgl})
        n127 = call "FitParametersRAW2Pixel.vi"("Pixel Size"=w251, "Subsampling"=w192, "ROI Offset"=w220, "Best Fits In"=w226) -> ("Fits metric"=w244:T3, "Fits Pixel"=w237:dbl[])  [unwired: 6 in]
        "Beam Parameters" <- w244
        "Gaus Param" <- w244
        "Fit Pixel" <- w237
        n128 = Unbundle By Name(w244) -> ("Width 1 (µm)"=w241:dbl, "Width 2 (µm)"=w240:dbl, "Amplitude (Counts)"=w242:dbl, "Position Max X(µm)"=w239:dbl, "Position Max Y(µm)"=w238:dbl)
        n129 = call "MajorMinorAxes.vi"("Best Fits"=w237, "Image in"=w245) -> ("cross lines"=→"Cross lines":T2)  [unwired: 8 in]
        n130 = call "EllipseOverlay.vi"("Fitted Parameters (Pixel)"=w237) -> ("Array"=→"Ellipse Points":cluster{"x out":dbl, "y out":dbl}[])  [unwired: 9 in]
        n131 = Cluster To Array(cluster=w244) -> (array=w252:dbl[])
        n132 = Build Array(w190, w226, w237, w252) -> (w253:dbl[][])
        n133 = Unbundle By Name(w204) -> ("status"=w205:bool)
        n134 = Transpose 2D Array(2D array=w253) -> (transposed array=→"parameter \narray":dbl[][])
        n135 = case shown="True" w205 {
          frame False {
          }
          frame True {
            n136 = property on="Cyclic\nCalculation" class="Bool (strict)"("Value"=FALSE ("Cyclic\nCalculation")) -> ()  [unwired: 2 in, 2 out]
          }
        }
        n137 = call "DurationTime.vi"("error in"=w204, "Starttime (Ticks in ms)"=w212) -> ("error out"=w224:errorcluster, "Time (ms)"=→"GausFit Time":u32)  [unwired: 8 in]
        n138 = Add(x=w241, y=w240) -> (x+y=w249:dbl)
        n139 = Bundle("Amplitude (Counts)"=w242, "Position Max X(µm)"=w239, "Position Max Y(µm)"=w238) -> (→"Beam Parameters\nfor Target":T19)  [unwired: 1 in]
        n140 = Divide(x=w240, y=w241) -> (x/y=→"Ellipticity":dbl)
        n141 = Divide(x=w249, y=2.0) -> (x/y=→"Mean \nRadius":dbl)
        n142 = local read "Show Target \nPoint Axes"() -> (w213:bool)
        n143 = property on="Gaussianfit" class="Bool (strict)"(error in=w224, "Value"=FALSE ("Gaussianfit 2")) -> (error out=w223:errorcluster)  [unwired: 1 in, 1 out]
        n144 = case shown="True" w213 {
          tunnel: w223 -> [w308 w310]
          tunnel: [w308 w309] -> w222
          frame False {
          }
          frame True {
            n145 = property on="Gaussian Fit completed" class="Bool (strict)"(error in=w310, "Val(Sgnl)"=TRUE ("Gaussian Fit completed")) -> (error out=w309:errorcluster)  [unwired: 1 in, 1 out]
          }
        }
      }
      event "Set Exposure": Value Change {
        n146 = event-data() -> ("Time"=w318:u32)  [unwired: 1 in, 5 out]
        n147 = local read "CAM\ninitialized"() -> (w321:bool)
        n148 = case shown="True" w321 {
          tunnel: w322 -> [w323 w330]
          tunnel: [w323 w329] -> w319
          tunnel: ["Camera not initialized, Press Start Camera" ("MainState") w328] -> w320
          frame False {
          }
          frame True {
            n149 = local read "Camera Handle"() -> (w331:T10)
            n150 = property class="IMAQdx"(reference=w331, error in=w330, "ActiveAttribute"="Exposure::Value", "ValueDBL"="Set: Exposure::Value") -> (error out=w329:errorcluster, "ValueDBL"=w327:dbl, "ValueString"=w325:string)  [unwired: 1 out]
            n151 = local write "Set: Exposure::Value"(w327) -> ()
            n152 = Concatenate Strings("Exposure time set to (s): " ("string"), w325) -> (w328:string)
          }
        }
      }
      event "Set Gain": Value Change {
        n153 = event-data() -> ("Time"=w334:u32)  [unwired: 1 in, 5 out]
        n154 = local read "CAM\ninitialized"() -> (w335:bool)
        n155 = case shown="True" w335 {
          tunnel: w338 -> [w339 w345]
          tunnel: [w339 w344] -> w337
          tunnel: ["Camera not initialized, Press Start Camera" ("MainState") w342] -> w336
          frame False {
          }
          frame True {
            n156 = local read "Camera Handle"() -> (w348:T10)
            n157 = property class="IMAQdx"(reference=w348, error in=w345, "ActiveAttribute"="Gain::Value", "ValueI64"="Set: Gain::Value") -> (error out=w344:errorcluster, "ValueI64"=w346:i64, "ValueString"=w341:string)  [unwired: 1 out]
            n158 = local write "Set: Gain::Value"(w346) -> ()
            n159 = Concatenate Strings("Exposure time set to (s): " ("string"), w341) -> (w342:string)
          }
        }
      }
      event "Exposure::Mode": Value Change {
        n160 = event-data() -> ("Time"=w352:u32)  [unwired: 1 in, 5 out]
        n161 = local read "CAM\ninitialized"() -> (w351:bool)
        n162 = case shown="True" w351 {
          tunnel: w354 -> [w355 w369]
          tunnel: [w355 w368] -> w353
          tunnel: ["Camera not initialized, Press Start Camera" ("MainState") "Exposure Mode set" ("MainState")] -> w350
          frame False {
          }
          frame True {
            n163 = local read "Camera Handle"() -> (w370:T10)
            n164 = case shown="0" "Exposure::Mode" {
              selector: "Exposure::Mode" -> [w373 w379 w386]
              tunnel: w370 -> [w377 w383 w388]
              tunnel: w369 -> [w376 w382 w387]
              tunnel: [w377 w383 w388] -> w366
              tunnel: [w376 w382 w387] -> w365
              tunnel: [w375 w379 w386] -> w364
              tunnel: [w372 T16."Disabled and Grayed Out" ("Disabled") T16."Enabled" ("Disabled")] -> w360
              tunnel: [w372 w378 w384] -> w358
              tunnel: [w372 w378 w384] -> w357
              frame 0 {
                w372 = T16."Disabled and Grayed Out" ("Disabled")
                w375 = u32 2 items=["Auto (Extended)", "Auto (Standard)", "Manual"] ("Exposure::Mode")
                # "good auto"
                n165 = local write "AutoAcquisitionState"(T8."idle" ("AutoAcquisitionState")) -> ()
                n166 = property on="Gain::Mode" class="Ring (strict)"("Value"=w373) -> ()  [unwired: 2 in, 2 out]
                n167 = property on="Enable AEC & AGC" class="Bool (strict)"("Value"=TRUE ("Enable AEC & AGC")) -> ()  [unwired: 2 in, 2 out]
              }
              frame 1 {
                w378 = T16."Enabled" ("Disabled")
                # "Auto"
                n168 = property on="Enable AEC & AGC" class="Bool (strict)"("Value"=FALSE ("Enable AEC & AGC")) -> ()  [unwired: 2 in, 2 out]
              }
              frame 2, Default {
                w384 = T16."Enabled" ("Disabled")
                # "manual"
                n169 = property on="Enable AEC & AGC" class="Bool (strict)"("Value"=FALSE ("Enable AEC & AGC")) -> ()  [unwired: 2 in, 2 out]
              }
            }
            n170 = property on="Gain::Mode" class="Ring (strict)"("DisabledEnum"=w358) -> ()  [unwired: 2 in, 2 out]
            n171 = property on="Set: Gain::Value" class="DigNum (strict)"("DisabledEnum"=w357) -> ()  [unwired: 2 in, 2 out]
            n172 = property on="Set Gain" class="Bool"("DisabledEnum"=w357) -> ()  [unwired: 2 in, 2 out]
            n173 = property class="IMAQdx"(reference=w366, error in=w365, "ActiveAttribute"="Exposure::Mode", "ValueU32"=w364) -> (error out=w362:errorcluster)  [unwired: 1 out]
            n174 = property on="Set Exposure" class="Bool"(error in=w362, "DisabledEnum"=w360) -> (error out=w361:errorcluster)  [unwired: 1 in, 1 out]
            n175 = property on="Set: Exposure::Value" class="DigNum (strict)"(error in=w361, "DisabledEnum"=w360) -> (error out=w368:errorcluster)  [unwired: 1 in, 1 out]
          }
        }
      }
      event "Gain::Mode": Value Change {
        n176 = event-data() -> ("Time"=w392:u32)  [unwired: 1 in, 5 out]
        n177 = local read "CAM\ninitialized"() -> (w391:bool)
        n178 = case shown="True" w391 {
          tunnel: w394 -> [w395 w407]
          tunnel: [w395 w406] -> w393
          tunnel: ["Camera not initialized, Press Start Camera" ("MainState") "Gain Mode Set" ("MainState")] -> w390
          frame False {
          }
          frame True {
            n179 = local read "Camera Handle"() -> (w408:T10)
            n180 = case shown="0" "Gain::Mode" {
              selector: "Gain::Mode" -> [w409 w415 w418]
              tunnel: w408 -> [w412 w417 w420]
              tunnel: w407 -> [w411 w416 w419]
              tunnel: [w412 w417 w420] -> w404
              tunnel: [w411 w416 w419] -> w403
              tunnel: [w410 w415 w418] -> w402
              tunnel: [T16."Disabled and Grayed Out" ("Disabled") T16."Disabled and Grayed Out" ("Disabled") T16."Enabled" ("Disabled")] -> w398
              frame 0 {
                w410 = u32 2 items=["Auto (Extended)", "Auto (Standard)", "Manual"] ("Gain::Mode")
                n181 = property on="Exposure::Mode" class="Ring (strict)"("Val(Sgnl)"=w409) -> ()  [unwired: 2 in, 2 out]
              }
              frame 1 {
                # "Auto"
              }
              frame 2, Default {
              }
            }
            n182 = property class="IMAQdx"(reference=w404, error in=w403, "ActiveAttribute"="Gain::Mode", "ValueU32"=w402) -> (error out=w399:errorcluster)  [unwired: 1 out]
            n183 = property on="Set Gain" class="Bool"(error in=w399, "DisabledEnum"=w398) -> (error out=w400:errorcluster)  [unwired: 1 in, 1 out]
            n184 = property on="Set: Gain::Value" class="DigNum (strict)"(error in=w400, "DisabledEnum"=w398) -> (error out=w406:errorcluster)  [unwired: 1 in, 1 out]
          }
        }
      }
      event "Record Background": Value Change {
        n185 = event-data() -> ("Time"=w426:u32)  [unwired: 1 in, 5 out]
        n186 = local read "CAM\ninitialized"() -> (w422:bool)
        n187 = local read "Streaming Started"() -> (w424:bool)
        n188 = And(x=w424, y=w422) -> (x .and. y?=w423:bool)
        n189 = case shown="False" w423 {
          tunnel: [w431 w432] -> w429
          tunnel: w428 -> [w431 w440]
          tunnel: ["Camera not initialized or stream not started" ("MainState") "Background recorded" ("MainState")] -> w427
          frame False {
          }
          frame True {
            # "Take care to deactivate background substraction before Capturing"
            n190 = property on="Subtract Background" class="Bool (strict)"(error in=w440, "Value"=FALSE ("Subtract Background")) -> (error out=w438:errorcluster)  [unwired: 1 in, 1 out]
            n191 = while {
              tunnel: [w451] -> w433
              tunnel: w438 -> [w451]
              stop <- w450 stop-if-true
              n192 = local read "Stream completed"() -> (w452:bool)
              n193 = Wait (ms)(milliseconds to wait=u32 100) -> ()  [unwired: 1 out]
              n194 = Not(x=w452) -> (.not. x?=w450:bool)
            }
            n195 = local read "IMAQ Background Image"() -> (w436:T4)
            n196 = local read "IMAQ Actual Image"() -> (w437:T4)
            n197 = flat-sequence {
              tunnel: w437 -> [w448]
              tunnel: w436 -> [w447]
              tunnel: [w446] -> w435
              tunnel: w433 -> [w445]
              tunnel: [w444] -> w434
              frame #0 {
                n198 = while {
                  stop <- w443 continue-if-true
                  n199 = property on="Image Busy" class="Bool (strict)"() -> ("Value"=w443:bool)  [unwired: 2 in, 2 out]
                }
              }
              frame #1 {
                n200 = call "IMAQ Copy"("error in (no error)"=w445, "Image Dst"=w447, "Image Src"=w448) -> ("error out"=w444:errorcluster, "Image Dst Out"=w446:T4)  [unwired: 3 in]
              }
            }
            n201 = property on="Subtract Background" class="Bool (strict)"(error in=w434, "Value"=TRUE ("Subtract Background")) -> (error out=w432:errorcluster)  [unwired: 1 in, 1 out]
            n202 = local write "Recorded Background"(w435) -> ()
            "Recorded Background" <- w435
          }
        }
        n203 = property on="Tab Control" class="TabCtl (strict)"("Value"=T17."Background" ("Tab Control")) -> ()  [unwired: 2 in, 2 out]
      }
      event "CalcHistogram": Value Change {
        n204 = event-data() -> ("Time"=w454:u32)  [unwired: 1 in, 5 out]
        n205 = local read "CAM\ninitialized"() -> (w453:bool)
        n206 = case shown="True" w453 {
          tunnel: ["Camera not initialized, Press Start Camera" ("MainState") w468] -> w457
          tunnel: [w458 w467] -> w456
          tunnel: w455 -> [w458 w466]
          frame False {
          }
          frame True {
            n207 = control-ref of="IMAQ Actual Image"() -> (w461:refnum<vi>)
            n208 = property on="Property Node" class="ImageControl"(reference=w461, error in=w466) -> (error out=w462:errorcluster, "ROI"=w465:T15)  [unwired: 1 out]
            n209 = Unbundle By Name(w465) -> ("Global Rectangle"=w464:i32[])
            n210 = property on="Tab Control" class="TabCtl (strict)"("Value"=T17."Histrogram" ("Tab Control")) -> ()  [unwired: 2 in, 2 out]
            n211 = Array Size(array=w464) -> (size(s)=w463:i32)
            n212 = case shown="1, Default" w463 {
              tunnel: [w469 w496] -> w467
              tunnel: w465 -> [_ w483]
              tunnel: ["No ROI selected" "Histogram"] -> w468
              tunnel: w462 -> [w470 w481]
              frame 0 {
                n213 = call "Display Message to User"("error in (no error)"=w470) -> ("error out"=w469:errorcluster)  [unwired: 9 in, 1 out]
              }
              frame 1, Default {
                w488 = 100.0  # Prozent
                w491 = 5 ("y")
                n214 = local read "IMAQ Actual Image"() -> (w474:T4)
                n215 = call "IMAQ Create"("Image Name"="MaskImage", "error in (no error)"=w481) -> ("New Image"=w497:T4, "error out"=w484:errorcluster)  [unwired: 3 in]
                n216 = call "IMAQ ROIToMask 2"("error in (no error)"=w484, "ROI Descriptor"=w483, "Image"=w497) -> ("error out"=w478:errorcluster, "Image Out"=w475:T4)  [unwired: 6 in, 1 out]
                n217 = flat-sequence {
                  tunnel: w478 -> [w504]
                  tunnel: [w503] -> w477
                  tunnel: w475 -> [w500]
                  tunnel: w474 -> [w501]
                  tunnel: [w500] -> w473
                  tunnel: [w505] -> w472
                  tunnel: [w502] -> w476
                  frame #0 {
                    n218 = while {
                      stop <- w499 continue-if-true
                      n219 = property on="Image Busy" class="Bool (strict)"() -> ("Value"=w499:bool)  [unwired: 2 in, 2 out]
                    }
                  }
                  frame #1 {
                    n220 = call "GetHistogram.vi"("Image"=w501, "Mask"=w500, "error in"=w504) -> ("Waveform Graph"=w505:u32[], "Gray Level Intensities"=w502:T6, "error out"=w503:errorcluster)  [unwired: 10 in]
                  }
                }
                n221 = local read "image width"() -> (w495:u16)
                n222 = local read "image heigth"() -> (w494:u16)
                n223 = Array Size(array=w472) -> (size(s)=w486:i32)
                n224 = Subtract(x=w486, y=w491) -> (x-y=w492:i32)
                n225 = Array Subset(array=w472, index=w492, length=w491) -> (w490:u32[])
                n226 = To Double Precision Float(number=w494) -> (double precision float=w479:dbl)
                n227 = To Double Precision Float(number=w495) -> (double precision float=w480:dbl)
                n228 = Add Array Elements(numeric array=w490) -> (sum=w485:u32)
                n229 = Multiply(x=w480, y=w479) -> (x*y=w493:dbl)
                n230 = Divide(x=w485, y=w493) -> (x/y=w489:dbl)
                n231 = Multiply(x=w489, y=w488) -> (x*y=→"Sättigung":dbl)
                n232 = call "Imaq Dispose"("Image"=w473, "error in (no error)"=w477) -> ("error out"=w496:errorcluster)  [unwired: 4 in]
                "Gray Level Intensities" <- w476
                "Histogramm of ROI" <- w472
              }
            }
          }
        }
      }
      event "stop", "Exit from Gaussian cycle", "Exit from Control refresh", "Exit from stream complete", "Exit from AGC/AEC": Value Change {
        n233 = event-data() -> ("Time"=w506:u32, "NewVal"=w512:bool)  [unwired: 1 in, 4 out]
        n234 = local read "CAM\ninitialized"() -> (w513:bool)
        n235 = case shown="True" w513 {
          tunnel: [w515 w521] -> w514
          tunnel: ["no cam initialized" w522] -> w511
          tunnel: w507 -> [w515 w520]
          frame False {
          }
          frame True {
            # "Dont Dispose Image \nto see the Image \nafter shutdown"
            n236 = local read "Streaming Started"() -> (w524:bool)
            n237 = local read "Camera Handle"() -> (w523:T10)
            n238 = flat-sequence {
              tunnel: w520 -> [w536]
              tunnel: w524 -> [w537]
              tunnel: w523 -> [w538]
              tunnel: [w538] -> w530
              tunnel: [w537] -> w529
              tunnel: [w536] -> w528
              tunnel: w530 -> [w541]
              tunnel: [w541] -> w527
              tunnel: w529 -> [w540]
              tunnel: [w540] -> w526
              tunnel: w528 -> [w539]
              tunnel: [w539] -> w525
              tunnel: [w546] -> w518
              tunnel: [w545] -> w522
              tunnel: w527 -> [w549]
              tunnel: w526 -> [w548]
              tunnel: w525 -> [w547]
              tunnel: [w544] -> w519
              frame #0 {
                n239 = local write "Streaming Started"(FALSE ("Streaming Started")) -> ()
              }
              frame #1 {
                n240 = while {
                  stop <- w542 stop-if-true
                  n241 = local read "Stream completed"() -> (w542:bool)
                }
              }
              frame #2 {
                n242 = case shown="False" w548 {
                  tunnel: w549 -> [w550 w556]
                  tunnel: w547 -> [w552 w555]
                  tunnel: [w552 w554] -> w546
                  tunnel: ["no stream running" ("MainState") "stream stopped" ("MainState")] -> w545
                  tunnel: [w550 w553] -> w544
                  frame False {
                  }
                  frame True {
                    n243 = call <vilib>:"IMAQdx Stop Acquisition.vi"("error in"=w555, "Session In"=w556) -> ("error out"=w557:errorcluster, "Session Out"=w558:T10)  [unwired: 8 out]
                    n244 = call <vilib>:"IMAQdx Unconfigure Acquisition.vi"("error in"=w557, "Session In"=w558) -> ("error out"=w554:errorcluster, "Session Out"=w553:T10)  [unwired: 8 out]
                    n245 = local write "Camera Handle"(w553) -> ()
                  }
                }
                n246 = local write "Exit from Eventloop"(TRUE) -> ()
              }
            }
            n247 = local write "CAM\ninitialized"(FALSE) -> ()
            n248 = call <vilib>:"IMAQdx Close Camera.vi"("error in"=w518, "Session In"=w519) -> ("error out"=w517:errorcluster)  [unwired: 9 out]
            n249 = disable-structure shown="Disabled" {
              disable-tunnel: w517 -> [w533 _]
              disable-tunnel: [w532 _] -> w521
              frame Disabled {
                n250 = local read "IMAQ Actual Image"() -> (w534:T4)
                n251 = call "Imaq Dispose"("Image"=w534, "error in (no error)"=w533) -> ("error out"=w532:errorcluster)  [unwired: 4 in]
              }
              frame Enabled {
              }
            }
          }
        }
        n252 = Concatenate Strings(w511, ", " ("string"), "Close Camera" ("MainState")) -> (w508:string)
      }
      event "3D Image": Value Change {
        n253 = event-data() -> ("Time"=w564:u32)  [unwired: 1 in, 5 out]
        n254 = local read "CAM\ninitialized"() -> (w563:bool)
        n255 = case shown="True" w563 {
          tunnel: w565 -> [w567 w571]
          tunnel: [w567 w570] -> w562
          tunnel: ["Camera not initialized, Press Start Camera" ("MainState") "3D Image updated" ("MainState")] -> w561
          frame False {
          }
          frame True {
            n256 = local read "IMAQ Actual Image"() -> (w574:T4)
            n257 = call "IMAQ Create"("Image Name"="3D Image") -> ("New Image"=w573:T4)  [unwired: 4 in, 1 out]
            n258 = flat-sequence {
              tunnel: "3D options" -> [w586]
              tunnel: "Direction (NW)" -> [w585]
              tunnel: w574 -> [w584]
              tunnel: w573 -> [w583]
              tunnel: 1 ("Size reduction") -> [w582]
              tunnel: w571 -> [w581]
              tunnel: [w580] -> w570
              tunnel: [w579] -> w569
              frame #0 {
                n259 = while {
                  stop <- w578 continue-if-true
                  n260 = property on="Image Busy" class="Bool (strict)"() -> ("Value"=w578:bool)  [unwired: 2 in, 2 out]
                }
              }
              frame #1 {
                n261 = call "IMAQ 3DView"("3D options"=w586, "Direction (NW)"=w585, "error in (no error)"=w581, "Size reduction"=w582, "Image Dst"=w583, "Image Src"=w584) -> ("error out"=w580:errorcluster, "Image Dst Out"=w579:T4)  [unwired: 4 in]
              }
            }
            "3D Image 2" <- w569
          }
        }
        n262 = property on="Tab Control" class="TabCtl (strict)"("Value"=T17."3D Image" ("Tab Control")) -> ()  [unwired: 2 in, 2 out]
      }
      event "Set Target Point": Value Change {
        n263 = event-data() -> ()  [unwired: 1 in, 6 out]
        n264 = local read "CAM\ninitialized"() -> (w588:bool)
        n265 = case shown="True" w588 {
          frame False {
          }
          frame True {
            n266 = local read "Cross lines"() -> (→"Target Point cross lines":T2)
            n267 = local read "Ellipse Points"() -> (→"Target Points Ellipse Points":cluster{"x out":dbl, "y out":dbl}[])
            n268 = local read "Beam Parameters"() -> (w592:T9)
            "Beam Parameters Target Point" <- w592
            n269 = Unbundle By Name(w592) -> ("Position X (µm)"=w596:dbl, "Position Y (µm)"=w595:dbl)
            n270 = Bundle By Name(cluster=T12 {"X"=0.0, "Y"=0.0} ("Point 2"), "X"=w596, "Y"=w595) -> (→"Point":T12)
            n271 = property on="Show Target \nPoint Axes" class="Bool (strict)"("Value"=TRUE ("Cyclic\nCalculation")) -> ()  [unwired: 2 in, 2 out]
            n272 = property on="Cyclic\nCalculation" class="Bool (strict)"("Value"=TRUE ("Cyclic\nCalculation")) -> ()  [unwired: 2 in, 2 out]
          }
        }
        n273 = property on="Tab Beam" class="TabCtl (strict)"("Value"=enum32{"Beam Parameters", "Navigate to Target"}."Navigate to Target" ("Tab Beam")) -> ()  [unwired: 2 in, 2 out]
      }
    }
    "error Event" <- w45
    "EventState" <- w55
    n274 = local write "Subtract Background"("Subtract Background") -> ()
    n275 = call "DurationTime.vi"("error in"=w45, "Starttime (Ticks in ms)"=w49) -> ("error out"=w46:errorcluster, "Time (ms)"=→"Time\nEvent(ms)":u32)  [unwired: 8 in]
    n276 = Unbundle By Name(w46) -> ("status"=w52:bool, "code"=w50:i32)
    n277 = call <vilib>:"General Error Handler.vi"("error in (no error)"=w46) -> ("error out"=w47:errorcluster)  [unwired: 10 in, 4 out]
    n278 = case shown="True" w52 {
      tunnel: w50 -> [_ w61]
      tunnel: w47 -> [w56 w58]
      tunnel: [w56 w60] -> w51
      frame False {
      }
      frame True {
        n279 = property on="Cyclic\nCalculation" class="Bool (strict)"(error in=w58, "Value"=FALSE ("Cyclic\nCalculation")) -> (error out=w57:errorcluster)  [unwired: 1 in, 1 out]
        n280 = call <vilib>:"Clear Errors.vi"("error in (no error)"=w57, "specific error code to clear (0: all)"=w61) -> ("error out"=w60:errorcluster)  [unwired: 4 in, 1 out]
      }
    }
  }
  "Exit from Eventloop" <- w27
  n281 = while {
    tunnel: [w600] -> w28
    shift-right: [w598] -> _
    shift-left: _ -> [w599]
    stop <- w600 stop-if-true
    n282 = event shown="[1] \"Next AEC & AGC iteration\": Value Change" {
      selector: _ -> [_ _ _]
      dyn-events: _ -> [_ _ _]
      timeout: _ -> [_ _ _]
      tunnel: [_ _ w726] -> w600
      tunnel: w599 -> [_ w602 _]
      tunnel: [_ w601 _] -> w598
      event Timeout {
        n283 = event-data() -> ()  [unwired: 1 in, 3 out]
      }
      event "Next AEC & AGC\niteration": Value Change {
        # "Reset"
        n284 = event-data() -> ()  [unwired: 1 in, 6 out]
        n285 = property on="Next AEC & AGC\niteration" class="Bool (strict)"("Value"=FALSE ("Next AEC & AGC\niteration")) -> ()  [unwired: 2 in, 2 out]
        n286 = stacked-sequence {
          seq-local: [w720 _ _] -> [_ _ w724]
          tunnel: [_ w721 _] -> w603
          frame #0 {
            n287 = call <vilib>:"High Resolution Relative Seconds.vi"() -> ("relative seconds"=w720:dbl)
          }
          frame #1 {
            n288 = local read "IMAQ Actual Image"() -> (w722:T4)
            n289 = call "IMAQ Histogram"("Image"=w722) -> ("Histogram Report"=w721:T1)  [unwired: 9 in, 1 out]
          }
          frame #2 {
            n290 = call <vilib>:"High Resolution Relative Seconds.vi"() -> ("relative seconds"=w725:dbl)
            n291 = Subtract(x=w725, y=w724) -> (x-y=→"Time\nAGC\nHist":dbl)
          }
        }
        "Histogram Report" <- w603
        n292 = Unbundle By Name(w603) -> ("Maximal Value"=w604:sgl)
        n293 = stacked-sequence {
          seq-local: [w606 _ _] -> [_ _ w718]
          tunnel: w604 -> [_ w610 _]
          tunnel: w602 -> [_ w608 _]
          tunnel: [_ w607 _] -> w601
          frame #0 {
            n294 = call <vilib>:"High Resolution Relative Seconds.vi"() -> ("relative seconds"=w606:dbl)
          }
          frame #1 {
            n295 = Divide(x=w610, y="Max Intensity") -> (x/y=→"ImgMax/Max":dbl)
            n296 = local read "Camera Handle"() -> (w614:T10)
            n297 = case shown="\"Find max gain\"" "AutoAcquisitionState" {
              tunnel: w614 -> [_ w627 w631 w645 w673 w678]
              tunnel: w610 -> [_ _ _ w636 _ w687]
              tunnel: "Max Intensity" -> [_ _ _ w637 _ _]
              tunnel: 0.3 ("y") -> [_ _ _ w638 _ _]
              tunnel: w608 -> [w615 w617 w629 w635 w671 w676]
              tunnel: [w615 w617 w629 w635 w671 w693] -> w607
              frame "idle", Default {
                # "Next State"
                n298 = property on="AutoAcquisitionState" class="Enum (strict)"("Value"=T8."init" ("AutoAcquisitionState")) -> ()  [unwired: 2 in, 2 out]
              }
              frame "init" {
                w618 = T16."Disabled and Grayed Out" ("Disabled")
                w621 = u32 2 items=["Auto"=1, "Manual"=2] ("Gain::Mode")
                # "Next State"
                n299 = local read "GValueMin"() -> (w619:dbl)
                n300 = local read "EValueMax"() -> (w625:dbl)
                n301 = Divide(x=w625, y=4.0) -> (x/y=w624:dbl)
                n302 = property class="IMAQdx"(reference=w627, "ActiveAttribute"="Exposure::Value", "ValueDBL"=w624, "ActiveAttribute"="Gain::Mode", "ValueU32"=w621, "ActiveAttribute"="Gain::Value", "ValueDBL"=w619) -> ()  [unwired: 1 in, 2 out]
                n303 = property on="Gain::Mode" class="Ring (strict)"("DisabledEnum"=w618) -> ()  [unwired: 2 in, 2 out]
                n304 = property on="Set Gain" class="Bool"("DisabledEnum"=w618) -> ()  [unwired: 2 in, 2 out]
                n305 = property on="Set: Gain::Value" class="DigNum (strict)"("DisabledEnum"=w618) -> ()  [unwired: 2 in, 2 out]
                n306 = property on="AutoAcquisitionState" class="Enum (strict)"("Value"=T8."Find max exposure" ("AutoAcquisitionState")) -> ()  [unwired: 2 in, 2 out]
              }
              frame "Wait before exposure" {
                # "Update Value"
                # "Next State"
                n307 = property class="IMAQdx"(reference=w631, "ActiveAttribute"="Exposure::Value") -> ("ValueDBL"=w630:dbl)  [unwired: 1 in, 2 out]
                n308 = property on="AutoAcquisitionState" class="Enum (strict)"("Value"=T8."Find max exposure" ("AutoAcquisitionState")) -> ()  [unwired: 2 in, 2 out]
                n309 = property on="Set: Exposure::Value" class="DigNum (strict)"("Value"=w630) -> ()  [unwired: 2 in, 2 out]
              }
              frame "Find max exposure" {
                # "Next Exposure"
                # "Annahme: Gain=0"
                n310 = local read "Set: Exposure::Value"() -> (w646:dbl)
                n311 = Multiply(x=w637, y=w638) -> (x*y=w639:dbl)
                n312 = Multiply(x=w637, y=0.8) -> (x*y=w640:dbl)
                n313 = call "CalcExposeWithoutSaturation.vi"("Actual Exposuretime"=w646, "Maximal Intensity that should not be reached"=w637, "Maximal Intensity in Image"=w636) -> ("New Exposuretime\nnext smaller"=w642:dbl)  [unwired: 1 in, 1 out]
                n314 = Less?(x=w636, y=w640) -> (x < y?=w643:bool)
                n315 = Less?(x=w639, y=w636) -> (x < y?=w644:bool)
                n316 = case shown="True" w644 {
                  tunnel: w645 -> [w651 w657]
                  tunnel: w642 -> [w650 _]
                  tunnel: w643 -> [_ w658]
                  tunnel: u32 2 ("y") -> [_ w656]
                  frame False {
                    # "i<i_max/2\nincrease exp"
                    n317 = local read "EValueMax"() -> (w649:dbl)
                    n318 = local read "EValueMin"() -> (w652:dbl)
                    n319 = In Range and Coerce(upper limit=w649, x=w650, lower limit=w652) -> (coerced(x)=w648:dbl)  [unwired: 1 out]
                    n320 = Equal?(x=w649, y=w648) -> (x = y?=w647:bool)
                    n321 = case shown="False" w647 {
                      frame True {
                        # "max exposure reached"
                        # "Next State"
                        n322 = property on="AutoAcquisitionState" class="Enum (strict)"("Value"=T8."Wait before gain" ("AutoAcquisitionState")) -> ()  [unwired: 2 in, 2 out]
                      }
                      frame False {
                        # "Next State"
                        n323 = property on="AutoAcquisitionState" class="Enum (strict)"("Value"=T8."Wait before exposure" ("AutoAcquisitionState")) -> ()  [unwired: 2 in, 2 out]
                      }
                    }
                    n324 = property class="IMAQdx"(reference=w651, "ActiveAttribute"="Exposure::Value", "ValueDBL"=w648) -> ()  [unwired: 1 in, 2 out]
                    n325 = property on="Set: Exposure::Value" class="DigNum (strict)"("Value"=w648) -> ()  [unwired: 2 in, 2 out]
                  }
                  frame True {
                    # "i_max/2 < i"
                    n326 = case shown="True" w658 {
                      tunnel: w657 -> [w665 _]
                      tunnel: w656 -> [w662 _]
                      frame False {
                        # "i > i_max\nsaturated"
                        n327 = property on="Set: Exposure::Value" class="DigNum (strict)"() -> ("Value"=w659:dbl)  [unwired: 2 in, 2 out]
                        n328 = local read "EValueMax"() -> (w666:dbl)
                        n329 = Divide(x=w659, y=w662) -> (x/y=w663:dbl)
                        n330 = local read "EValueMin"() -> (w660:dbl)
                        n331 = Equal?(x=w659, y=w660) -> (x = y?=w661:bool)
                        n332 = case shown="True" w661 {
                          frame False {
                            # "Next State"
                            n333 = property on="AutoAcquisitionState" class="Enum (strict)"("Value"=T8."Wait before exposure" ("AutoAcquisitionState")) -> ()  [unwired: 2 in, 2 out]
                          }
                          frame True {
                            # "Next State"
                            n334 = property on="AutoAcquisitionState" class="Enum (strict)"("Value"=T8."Wait before gain" ("AutoAcquisitionState")) -> ()  [unwired: 2 in, 2 out]
                          }
                        }
                        n335 = In Range and Coerce(upper limit=w666, x=w663, lower limit=w660) -> (coerced(x)=w664:dbl)  [unwired: 1 out]
                        n336 = property class="IMAQdx"(reference=w665, "ActiveAttribute"="Exposure::Value", "ValueDBL"=w664) -> ()  [unwired: 1 in, 2 out]
                        n337 = property on="Set: Exposure::Value" class="DigNum (strict)"("Value"=w664) -> ()  [unwired: 2 in, 2 out]
                      }
                      frame True {
                        # "Next State"
                        # "i_max/2 < i < i_max"
                        # "optimal exposure found\ngo to GainControl"
                        n338 = property on="AutoAcquisitionState" class="Enum (strict)"("Value"=T8."Wait before gain" ("AutoAcquisitionState")) -> ()  [unwired: 2 in, 2 out]
                      }
                    }
                  }
                }
              }
              frame "Wait before gain" {
                # "Update Value"
                # "Next State"
                n339 = property class="IMAQdx"(reference=w673, "ActiveAttribute"="Gain::Value") -> ("ValueI64"=w672:i64)  [unwired: 1 in, 2 out]
                n340 = property on="AutoAcquisitionState" class="Enum (strict)"("Value"=T8."Find max gain" ("AutoAcquisitionState")) -> ()  [unwired: 2 in, 2 out]
                n341 = property on="Set: Gain::Value" class="DigNum (strict)"("Value"=w672) -> ()  [unwired: 2 in, 2 out]
              }
              frame "Find max gain" {
                # "Totbereich"
                # "Regelstruktur: I-Regler\nDer Integratorwert wird über das Schieberegister der äußeren While-Scheife dargestellt"
                # "Time not\nnomalized"
                # "|| exit if \nG>Max &&\nExp < max"
                # "exit if \nG<min &&\nExp > min"
                n342 = property on="Set: Exposure::Value" class="DigNum (strict)"() -> ("Value"=w682:dbl)  [unwired: 2 in, 2 out]
                n343 = local read "EValueMax"() -> (w684:dbl)
                n344 = local read "EValueMin"() -> (w683:dbl)
                n345 = Subtract(x="soll", y=w687) -> (x-y=w700:dbl)
                n346 = case shown="..-9" w700 {
                  selector: w700 -> [w711 _ w715]
                  tunnel: [w712 0.0 ("y") w716] -> w689
                  tunnel: 8.0 ("y") -> [w710 _ w714]
                  frame ..-9 {
                    n347 = Add(x=w711, y=w710) -> (x+y=w712:dbl)
                  }
                  frame -8..8, Default {
                  }
                  frame 9.. {
                    n348 = Subtract(x=w715, y=w714) -> (x-y=w716:dbl)
                  }
                }
                n349 = Not Equal?(x=w682, y=w683) -> (x != y?=w680:bool)
                n350 = Not Equal?(x=w682, y=w684) -> (x != y?=w681:bool)
                n351 = Less Than 0?(x=w689) -> (x < 0?=w699:bool)
                n352 = Multiply(x="1/T", y=w689) -> (x*y=w694:dbl)
                n353 = Greater Than 0?(x=w689) -> (x > 0?=w690:bool)
                n354 = local read "GValueMax"() -> (w679:dbl)
                n355 = local read "GValueMin"() -> (w686:dbl)
                n356 = Greater Or Equal?(x=w676, y=w679) -> (x >= y?=w691:bool)
                n357 = Less Or Equal?(x=w676, y=w686) -> (x <= y?=w692:bool)
                n358 = Compound Arithmetic op=AND(w692, w699, w680) -> (w696:bool)
                n359 = Compound Arithmetic op=AND(w691, w690, w681) -> (w697:bool)
                n360 = Add(x=w694, y=w676) -> (x+y=w703:dbl)
                n361 = Or(x=w696, y=w697) -> (x .or. y?=w695:bool)
                n362 = In Range and Coerce(upper limit=w679, x=w703, lower limit=w686) -> (coerced(x)=w688:dbl)  [unwired: 1 out]
                "iValue" <- w688
                "iValue\nChart" <- w688
                n363 = case shown="True" w695 {
                  tunnel: w688 -> [w705 _]
                  tunnel: [w705 16.0 ("upper limit")] -> w693
                  tunnel: [w705 i64 0 ("ValueI64")] -> w677
                  frame False {
                    # "Stay in state"
                    n364 = property on="AutoAcquisitionState" class="Enum (strict)"("Value"=T8."Wait before gain" ("AutoAcquisitionState")) -> ()  [unwired: 2 in, 2 out]
                  }
                  frame True {
                    # "True means\nExit to Exposure"
                    # "Reset Integrator,\nbut dont to 0 \nto prevent exit in \nnext gain-loop"
                    # "Next State"
                    n365 = property on="AutoAcquisitionState" class="Enum (strict)"("Value"=T8."Wait before exposure" ("AutoAcquisitionState")) -> ()  [unwired: 2 in, 2 out]
                  }
                }
                n366 = property class="IMAQdx"(reference=w678, "ActiveAttribute"="Gain::Value", "ValueI64"=w677) -> ("ValueI64"=w698:i64)  [unwired: 1 in, 2 out]
                n367 = property on="Set: Gain::Value" class="DigNum (strict)"("Value"=w698) -> ()  [unwired: 2 in, 2 out]
                "ist" <- w687
              }
            }
            "State" <- "AutoAcquisitionState"
          }
          frame #2 {
            n368 = call <vilib>:"High Resolution Relative Seconds.vi"() -> ("relative seconds"=w719:dbl)
            n369 = Subtract(x=w719, y=w718) -> (x-y=→"Time\nAGC/AEC\ncycle":dbl)
          }
        }
      }
      event "Exit from Eventloop": Value Change {
        n370 = event-data() -> ()  [unwired: 1 in, 6 out]
        n371 = local read "Exit from stream complete"() -> (w728:bool)
        n372 = local read "Exit from Control refresh"() -> (w729:bool)
        n373 = local read "Exit from Gaussian cycle"() -> (w730:bool)
        n374 = local read "Exit from Eventloop"() -> (w727:bool)
        n375 = Compound Arithmetic op=OR(w727, w728, w729, w730) -> (w726:bool)
      }
    }
  }
  "Exit from AGC/AEC" <- w28
  n376 = while {
    shift-right: [w731] -> _
    shift-left: "error in" -> [w733]
    tunnel: [w732] -> w26
    stop <- w732 stop-if-true
    n377 = stacked-sequence {
      seq-local: [w734 _ _] -> [_ _ w825]
      tunnel: w733 -> [_ w738 _]
      tunnel: [_ w736 _] -> w731
      tunnel: [_ w737 _] -> w732
      frame #0 {
        n378 = call <vilib>:"High Resolution Relative Seconds.vi"() -> ("relative seconds"=w734:dbl)
      }
      frame #1 {
        n379 = local read "Streaming Started"() -> (w743:bool)
        n380 = local read "CAM\ninitialized"() -> (w742:bool)
        n381 = And(x=w743, y=w742) -> (x .and. y?=w744:bool)
        n382 = case shown="True" w744 {
          tunnel: [w751 w788] -> w736
          tunnel: w738 -> [w751 w791]
          tunnel: [TRUE w787] -> w739
          frame False {
            n383 = Wait (ms)(milliseconds to wait=u32 100) -> ()  [unwired: 1 out]
          }
          frame True {
            w766 = 5 items=["Red", "Green", "Blue", "Hue", "Saturation", "Luminance", "Value", "Intensity"] ("Color Plane")
            w768 = T14 5 items=["Grayscale (U8)", "Grayscale (I16)", "Grayscale (SGL)", "Complex (CSG)", "RGB (U32)", "HSL (U32)", "RGB (U64)"] ("Image Type")
            w785 = IMAQdx_Buffer_Number_Mode."Next"  # Buffer Number  Mode
            w787 = TRUE ("Stream completed")
            # "release image"
            # "Indicate to other functions\nto wait"
            # "Show Image\nin display"
            # "Trigger AEC/AGC"
            # "Overlay target"
            # "Overlay target"
            # "Overlay Fit"
            # "Background Image"
            # "Convert RGB to Luminance\n(Grauwert Bild)"
            # "Get Image"
            # "Choose 'Next' as Buffer Mode,\nIn 'Last' Mode it does not wait \nfor the next image and one image \nis transmitted many times until \nthe next is captured"
            # "Video frame"
            n384 = local read "IMAQ Actual Image (RGB)"() -> (w782:T4)
            n385 = property on="Stream completed" class="Bool (strict)"(error in=w791, "Value"=FALSE ("Stream completed")) -> (error out=w790:errorcluster)  [unwired: 1 in, 1 out]
            n386 = local read "Camera Handle"() -> (w783:T10)
            n387 = call <vilib>:"IMAQdx Get Image2.vi"("Buffer Number Mode (Next)"=w785, "error in"=w790, "Image In"=w782, "Session In"=w783) -> ("error out"=w761:errorcluster, "Buffer Number Out"=w786:u32, "Image Out"=w762:T4)  [unwired: 4 in, 1 out]
            "Buffer Number" <- w786
            n388 = call <vilib>:"Calculate Frames per Second.vi"("Buffer Number"=w786) -> ("Processed Frames/s"=→"Frame Rate":dbl)  [unwired: 8 in, 2 out]
            n389 = local write "IMAQ Actual Image (RGB)"(w762) -> ()
            n390 = call "IMAQ Cast Image"("Image Type"=w768, "error in (no error)"=w761, "Image Src"=w762) -> ("error out"=w760:errorcluster, "Image Dst Out"=w767:T4)  [unwired: 7 in]
            n391 = local read "IMAQ Actual Image"() -> (w763:T4)
            n392 = property on="Image \nBusy" class="Bool (strict)"(error in=w760, "Value"=TRUE ("Image Busy")) -> (error out=w759:errorcluster)  [unwired: 1 in, 1 out]
            n393 = call "IMAQ ExtractSingleColorPlane"("Color Plane"=w766, "error in (no error)"=w759, "Image Dst"=w763, "Image Src"=w767) -> ("error out"=w765:errorcluster, "Image Dst Out"=w764:T4)  [unwired: 6 in]
            n394 = local read "Subtract Background"() -> (w781:bool)
            n395 = case shown="True" w781 {
              tunnel: w764 -> [w818 w823]
              tunnel: [w818 w819] -> w780
              tunnel: w765 -> [w817 w821]
              tunnel: [w817 w820] -> w779
              frame False {
              }
              frame True {
                n396 = local read "IMAQ Background Image"() -> (w822:T4)
                n397 = call "IMAQ Subtract"("Image Src A"=w823, "Image Dst"=w823, "Image Src B"=w822, "error in (no error)"=w821) -> ("Image Dst Out"=w819:T4, "error out"=w820:errorcluster)  [unwired: 3 in]
              }
            }
            n398 = case shown="True" "Show Axes Overlay" {
              tunnel: w780 -> [w808 w816]
              tunnel: w779 -> [w807 w815]
              tunnel: [w808 w812] -> w756
              tunnel: [w807 w814] -> w755
              frame False {
              }
              frame True {
                n399 = local read "Cross lines"() -> (w813:T2)
                n400 = call "MMAxesOverlay.vi"("error in (no error)"=w815, "cross lines"=w813, "Image in"=w816) -> ("error out"=w814:errorcluster, "Image out"=w811:T4)  [unwired: 7 in]
                n401 = local read "Ellipse Points"() -> (w810:cluster{"x out":dbl, "y out":dbl}[])
                n402 = call "IMAQ Overlay Multiple Lines 2"("Image"=w811, "Line End Points"=w810, "Color"=u32 15748608) -> ("Image Out"=w812:T4)  [unwired: 11 in, 1 out]
              }
            }
            n403 = case shown="True" "Show Target \nPoint Axes" {
              tunnel: w756 -> [w793 w801]
              tunnel: w755 -> [w792 w795]
              tunnel: [w793 w798] -> w758
              tunnel: [w792 w800] -> w757
              frame False {
              }
              frame True {
                w794 = u32 8947848 ("Color Major")
                n404 = local read "Target Point cross lines"() -> (w799:T2)
                n405 = call "MMAxesOverlay.vi"("Color Minor"=w794, "Color Major"=w794, "error in (no error)"=w795, "cross lines"=w799, "Image in"=w801) -> ("error out"=w800:errorcluster, "Image out"=w797:T4)  [unwired: 5 in]
                n406 = local read "Target Points Ellipse Points"() -> (w796:cluster{"x out":dbl, "y out":dbl}[])
                n407 = call "IMAQ Overlay Multiple Lines 2"("Image"=w797, "Line End Points"=w796, "Color"=w794) -> ("Image Out"=w798:T4)  [unwired: 11 in, 1 out]
              }
            }
            n408 = Not(x="Next AEC & AGC\niteration") -> (.not. x?=w769:bool)
            n409 = And(x="Enable AEC & AGC", y=w769) -> (x .and. y?=w770:bool)
            n410 = case shown="True" w770 {
              selector: w770 -> [_ w804]
              tunnel: [w803 w806] -> w774
              tunnel: w758 -> [w803 w806]
              tunnel: [w802 w805] -> w773
              tunnel: w757 -> [w802 w805]
              frame False {
              }
              frame True {
                n411 = property on="Next AEC & AGC\niteration" class="Bool (strict)"("Val(Sgnl)"=w804) -> ()  [unwired: 2 in, 2 out]
              }
            }
            n412 = property on="IMAQ Actual Image" class="ImageControl"(error in=w773, "Value"=w774) -> (error out=w776:errorcluster)  [unwired: 1 in, 1 out]
            n413 = property on="Image Busy" class="Bool (strict)"(error in=w776, "Value"=FALSE ("Image Busy")) -> (error out=w775:errorcluster)  [unwired: 1 in, 1 out]
            n414 = property on="Stream \ncompleted" class="Bool (strict)"(error in=w775, "Value"=w787) -> (error out=w788:errorcluster)  [unwired: 1 in, 1 out]
          }
        }
        "Stream error out" <- w736
        n415 = local read "Exit from stream complete"() -> (w747:bool)
        n416 = local read "Exit from Control refresh"() -> (w746:bool)
        n417 = local read "Exit from Gaussian cycle"() -> (w745:bool)
        n418 = local read "Exit from Eventloop"() -> (w748:bool)
        n419 = local read "Exit from AGC/AEC"() -> (w735:bool)
        n420 = call <vilib>:"General Error Handler.vi"("error in (no error)"=w736) -> ()  [unwired: 10 in, 5 out]
        n421 = Unbundle By Name(w736) -> ("status"=w740:bool)
        n422 = Compound Arithmetic op=OR(w735, w748, w747, w746, w745) -> (w749:bool)
        n423 = Or(x=w740, y=w749) -> (x .or. y?=w737:bool)
        n424 = Or(x=w739, y=w737) -> (x .or. y?=→"Stream completed":bool)
      }
      frame #2 {
        # "Stacked sequence structure\nto measure the acquisitiontime"
        n425 = call <vilib>:"High Resolution Relative Seconds.vi"() -> ("relative seconds"=w826:dbl)
        n426 = Subtract(x=w826, y=w825) -> (x-y=→"Time\nAcqisition(s)" →"AcquisitionTime":dbl)
      }
    }
  }
  "Exit from stream complete" <- w26
  n427 = local write "Streaming Started"(FALSE ("Exited from stream")) -> ()
  n428 = local write "Stream completed"(TRUE ("Exited from stream")) -> ()
  n429 = local write "CAM\ninitialized"(FALSE ("Exited from stream")) -> ()
  n430 = local write "Subtract Background"(FALSE ("Cyclic \nRecalculation")) -> ()
  n431 = local write "Gaussian Fit completed"(FALSE ("Gaussianfit")) -> ()
  n432 = while {
    tunnel: [w827] -> w23
    stop <- w827 stop-if-true
    n433 = event shown="[1] \"Gaussian Fit completed\": Value Change" {
      selector: _ -> [_ _ _]
      dyn-events: _ -> [_ _ _]
      timeout: _ -> [_ _ _]
      tunnel: [_ _ w858] -> w827
      event Timeout {
        n434 = event-data() -> ()  [unwired: 1 in, 3 out]
      }
      event "Gaussian Fit completed": Value Change {
        n435 = event-data() -> ()  [unwired: 1 in, 6 out]
        n436 = local read "Show Target \nPoint Axes"() -> (w840:bool)
        n437 = case shown="True" w840 {
          frame False {
          }
          frame True {
            n438 = local read "Beam Parameters Target Point"() -> (w857:T9)
            n439 = local read "Beam Parameters"() -> (w856:T9)
            n440 = Negate(x="Threshold (µm)") -> (-x=w845:dbl)
            n441 = Negate(x="Threshold (µm)") -> (-x=w846:dbl)
            n442 = Unbundle By Name(w857) -> ("Position X (µm)"=w855:dbl, "Position Y (µm)"=w852:dbl)
            n443 = Unbundle By Name(w856) -> ("Position X (µm)"=w854:dbl, "Position Y (µm)"=w853:dbl)
            n444 = Subtract(x=w854, y=w855) -> (x-y=w841:dbl)
            "dx" <- w841
            n445 = Less?(x=w841, y=w845) -> (x < y?=w851:bool)
            "right" <- w851
            n446 = Greater?(x=w841, y="Threshold (µm)") -> (0:w850:bool)
            "left" <- w850
            n447 = Subtract(x=w853, y=w852) -> (x-y=w842:dbl)
            "dy" <- w842
            n448 = Less?(x=w842, y=w846) -> (x < y?=w849:bool)
            "down" <- w849
            n449 = Greater?(x=w842, y="Threshold (µm)") -> (0:w848:bool)
            "up" <- w848
            n450 = Compound Arithmetic op=OR(w851, w850, w849, w848) -> (invert →"center":bool)
            n451 = property on="Gaussian Fit completed" class="Bool (strict)"("Value"=FALSE ("Gaussian Fit completed")) -> ()  [unwired: 2 in, 2 out]
          }
        }
        n452 = local read "Point"() -> (w829:T12)
        n453 = local read "Beam Parameters"() -> (w828:T9)
        n454 = Unbundle By Name(w828) -> ("Position X (µm)"=w830:dbl, "Position Y (µm)"=w832:dbl)
        n455 = Unbundle By Name(w829) -> ("X"=w831:sgl, "Y"=w833:sgl)
        n456 = Subtract(x=w830, y=w831) -> (x-y=w834:dbl)
        n457 = Subtract(x=w832, y=w833) -> (x-y=w835:dbl)
        n458 = Square(x=w834) -> (x^2=w836:dbl)
        n459 = Square(x=w835) -> (x^2=w837:dbl)
        n460 = Add(x=w836, y=w837) -> (x+y=w838:dbl)
        n461 = Square Root(x=w838) -> (sqrt(x)=→"Absolute Distance (µm)":dbl)
      }
      event "Exit from Eventloop": Value Change {
        n462 = event-data() -> ()  [unwired: 1 in, 6 out]
        n463 = local read "Exit from stream complete"() -> (w860:bool)
        n464 = local read "Exit from Control refresh"() -> (w861:bool)
        n465 = local read "Exit from Gaussian cycle"() -> (w862:bool)
        n466 = local read "Exit from Eventloop"() -> (w859:bool)
        n467 = local read "Exit from AGC/AEC"() -> (w863:bool)
        n468 = Compound Arithmetic op=OR(w863, w859, w860, w861, w862) -> (w858:bool)
      }
    }
  }
  "Exit from Target Point" <- w23
  n469 = local write "AutoAcquisitionState"(T8."idle" ("AutoAcquisitionState")) -> ()
  n470 = local write "Enable AEC & AGC"(TRUE ("Enable AEC & AGC")) -> ()
  n471 = local write "Next AEC & AGC\niteration"(FALSE ("Next AEC & AGC\niteration")) -> ()
  n472 = property on="Exit from Eventloop" class="Bool (strict)"("Val(Sgnl)"=w27) -> ()  [unwired: 2 in, 2 out]
  n473 = property on="Streaming Started" class="Bool (strict)"(error in=w33, "Value"=FALSE ("Streaming Started")) -> ()  [unwired: 1 in, 2 out]
  n474 = property on="Exit from stream complete" class="Bool (strict)"("Val(Sgnl)"=w26) -> ()  [unwired: 2 in, 2 out]
  n475 = while {
    shift-right: [w877] -> _
    shift-left: "error in" -> [w878]
    tunnel: [w876] -> w31
    stop <- w876 stop-if-true
    n476 = local read "CAM\ninitialized"() -> (w879:bool)
    n477 = case shown="True" w879 {
      tunnel: [w882 w886] -> w877
      tunnel: w878 -> [w882 w887]
      frame False {
      }
      frame True {
        n478 = local read "Camera Handle"() -> (w888:T10)
        n479 = call "GetActualCameraParameters.vi"("Refnum in"=w888, "error in (no error)"=w887) -> ("ExposureValue"=→"ActValue:Exposure":string, "GainValue"=→"ActVal:Gain":string, "InverseExposureValue"=→"ActValue:InverseExposure":dbl, "error out"=w886:errorcluster)  [unwired: 8 in, 2 out]
      }
    }
    "error\nControl\nrefresh" <- w877
    n480 = property on="IMAQ Actual Image" class="ImageControl"() -> ("ZoomInteger"=w869:cluster{"X":i32, "Y":i32})  [unwired: 2 in, 2 out]
    n481 = property on="Differece Image to Ideal Gaussian" class="ImageControl"() -> ("ZoomInteger"=w868:cluster{"X":i32, "Y":i32})  [unwired: 2 in, 2 out]
    n482 = Wait (ms)(milliseconds to wait=u32 1000) -> ()  [unwired: 1 out]
    n483 = Not Equal?(x=w869, y=w868) -> (x != y?=w866:cluster{"X":bool, "Y":bool})
    n484 = Unbundle By Name(w866) -> ("X"=w865:bool)
    n485 = And(x="DualZoom", y=w865) -> (x .and. y?=w864:bool)
    n486 = case shown="True" w864 {
      tunnel: w869 -> [_ w881]
      frame False {
      }
      frame True {
        n487 = property on="Differece Image to Ideal Gaussian" class="ImageControl"("ZoomInteger"=w881) -> ()  [unwired: 2 in, 2 out]
      }
    }
    n488 = local read "Exit from stream complete"() -> (w874:bool)
    n489 = local read "Exit from Control refresh"() -> (w873:bool)
    n490 = local read "Exit from Gaussian cycle"() -> (w872:bool)
    n491 = local read "Exit from Eventloop"() -> (w875:bool)
    n492 = local read "Exit from AGC/AEC"() -> (w870:bool)
    n493 = Compound Arithmetic op=OR(w875, w874, w873, w872, w870) -> (w871:bool)
    n494 = local write "error Event"(w877) -> ()
    n495 = Or(x=w877, y=w871) -> (x .or. y?=w876:bool)
  }
  "Exit from Control refresh" <- w31
  n496 = while {
    tunnel: [w889] -> w30
    stop <- w889 stop-if-true
    n497 = flat-sequence {
      tunnel: [w900] -> w889
      frame #0 {
        n498 = First Call?() -> (First Call?: T/F=w897:bool)
        n499 = local read "Streaming Started"() -> (w891:bool)
        n500 = Not(x=w897) -> (.not. x?=w895:bool)
        n501 = Compound Arithmetic op=AND("Cyclic\nCalculation", w895, w891) -> (w894:bool)
        n502 = property on="Gaussianfit" class="Bool (strict)"() -> ("Value"=w890:bool)  [unwired: 2 in, 2 out]
        n503 = Not(x=w890) -> (.not. x?=w893:bool)
        n504 = And(x=w894, y=w893) -> (x .and. y?=w892:bool)
        n505 = case shown="True" w892 {
          frame False {
          }
          frame True {
            n506 = property on="Gaussianfit" class="Bool (strict)"("Val(Sgnl)"=TRUE ("Value (Signaling)")) -> ()  [unwired: 2 in, 2 out]
          }
        }
      }
      frame #1 {
        n507 = local read "Exit from stream complete"() -> (w902:bool)
        n508 = local read "Exit from Control refresh"() -> (w903:bool)
        n509 = local read "Exit from Gaussian cycle"() -> (w904:bool)
        n510 = local read "Exit from Eventloop"() -> (w901:bool)
        n511 = local read "Exit from AGC/AEC"() -> (w899:bool)
        n512 = Wait Until Next ms Multiple(millisecond multiple="Cycletime Task\nGaussian Fit") -> ()  [unwired: 1 out]
        n513 = Compound Arithmetic op=OR(w901, w902, w903, w904, w899) -> (w900:bool)
      }
    }
  }
  "Exit from Gaussian cycle" <- w30
  n514 = disable-structure shown="Disabled" {
    frame Disabled {
      n515 = local write "Cyclic\nCalculation"(FALSE ("Cyclic \nRecalculation")) -> ()
    }
    frame Enabled {
    }
  }
  n516 = local write "Exit from Eventloop"(w22) -> ()
  n517 = local write "Exit from stream complete"(w22) -> ()
  n518 = local write "Exit from Control refresh"(w22) -> ()
  n519 = local write "Exit from Gaussian cycle"(w22) -> ()
  n520 = local write "Exit from AGC/AEC"(w22) -> ()
  n521 = local write "Exit from Target Point"(w22) -> ()
